vi "EditorEinfachPC.vi"() -> ()   [LabVIEW 2010]
panel:
  in  "EinstellungenSpeichern":bool
  out "Spannung Mach":fxp<+/-,16,4> format="%.14g"
  in  "Temperatur Mach":dbl
  out "Spannung Trap":fxp<+/-,16,4> format="%.14g"
  in  "Temperatur Trap":dbl
  out "LangsameHeizungen":string[](array[string])
  in  "AllesSpeichern":bool
  in  "ModuleLH":i32[](array[numeric]) min=1 max=3 step=1
  in  "NamenLangsameHeizungen":string[](array[string])
  out "Schnelle Heizungen":string[](array[string])
  in  "Modul3/AIsNamen":string[](array[string])
  in  "Modul2/AIsNamen":string[](array[string])
  in  "Modul1/AIsNamen":string[](array[string])
  out "Methoden":T1(array[cluster]) {"FPGAPID"."proportional gain (Kc)" format="%.11g"; "FPGAPID"."integral gain (Kc*Ts/Ti)" format="%.11g"; "FPGAPID"."derivative gain (Kc*Td/Ts)" format="%.11g"; "FPGAFixp" format="%.14g"}
  in  "Methodenname":string
  in  "Int.Stop2":dbl
  in  "Int.Start2":dbl
  in  "Int.Stop1":dbl
  in  "Int.Start1":dbl
  in  "ZeitpktMS-2":dbl
  in  "ZeitpktMS-1":dbl
  in  "SPMPV":i32[](array[numeric])
  in  "ZeitpunkteMPV":dbl[](array[numeric])
  in  "Regler für den Probenfluß":i32
  in  "DateinameECD2":string
  in  "DateiordnerECD2":path
  in  "DateinameECD1":string
  in  "DateiordnerECD1":path
  in  "Wert2":dbl
  in  "Vergleichsoperator2":dbl(ring) items=["<", "<=", "=", ">=", ">", "=/="]
  in  "AbfragbareVariablen2":dbl(ring) items=["T-Trap1", "T-Trap2", "T-Stirling", "T-PreCol1", "T-PreCol2", "T-MainCol1", "T-MainCol2", "T-MainCol3", "T-MainCol4", "T-Bronkh1", "T-Bronkh2", "T-Bronkh3", "T-Bronkh4", "T-Valve2", "T-Oven", "T-Valve1", "T-TransfLine", "T-TurboPump", "T-StirlingPlatine", "T-Spare3", "T-Spare4", "T-Spare5", "T-Spare6", "MFM1-1", "MFM1-2", "P-HighPress", "P-LowPress", "P-Vac", "TurboSpeed", "I-AC", "I-Trap1", "I-Trap2", "Mod2/AI0", "Mod2/AI1", "Mod2/AI2", "Mod2/AI3", "Mod2/AI4", "Mod2/AI5", "Mod2/AI6", "Mod2/AI7", "Mod2/AI8", "Mod2/AI9", "Mod2/AI10", "Mod2/AI11", "Mod2/AI12", "Mod2/AI13", "Mod2/AI14", "Mod2/AI15", "Mod2/AI16", "Mod2/AI17", "Mod2/AI18", "Mod2/AI19", "Mod2/AI20", "Mod2/AI21", "Mod2/AI22", "Mod2/AI23", "Mod2/AI24", "Mod2/AI25", "Mod2/AI26", "Mod2/AI27", "Mod2/AI28", "Mod2/AI29", "Mod2/AI30", "Mod2/AI31", "Mod3/AI0", "Mod3/AI1", "Mod3/AI2", "Mod3/AI3", "Mod3/AI4", "Mod3/AI5", "Mod3/AI6", "Mod3/AI7", "Mod3/AI8", "Mod3/AI9", "Mod3/AI10", "Mod3/AI11", "Mod3/AI12", "Mod3/AI13", "Mod3/AI14", "Mod3/AI15", "Mod3/AI16", "Mod3/AI17", "Mod3/AI18", "Mod3/AI19", "Mod3/AI20", "Mod3/AI21", "Mod3/AI22", "Mod3/AI23", "Mod3/AI24", "Mod3/AI25", "Mod3/AI26", "Mod3/AI27", "Mod3/AI28", "Mod3/AI29", "Mod3/AI30", "Mod3/AI31", "WiderstTrap1", "TempTrap1", "WiderstTrap2", "TempTrap2", "TempMach1", "TempMach2", "Regler18"]
  in  "Dateiname Housekeeping":string
  in  "Dateiordner Housekeeping":path=path "C:/Users/Atmos/Desktop/Johnny"
  in  "Startmethode":i32=1
  in  "Dateien fürs MS schicken?":bool
  in  "Zwangsbedingungen":dbl[][](array[numeric])
  out "ZwangsBedingungen":string[][](array[string])
  in  "löschen":bool
  in  "Bedingung Nr. X":i32
  in  "Bedingung übernehmen":bool
  in  "Ausgangswert":dbl
  in  "BedienbareVariablen":dbl(ring) items=["Mod5/DIO5", "Mod5/DIO6", "Mod5/DIO7", "Mod5/DIO10", "Mod5/DIO11", "Mod5/DIO14", "Mod5/DIO15", "Mod5/DIO16", "Mod5/DIO17", "Mod5/DIO18", "Mod5/DIO20", "Mod5/DIO23", "Mod5/DIO25", "Mod5/DIO26", "Mod5/DIO27", "Mod5/DIO28", "Mod5/DIO29", "Mod5/DIO30", "Mod6/DIO0", "Mod6/DIO1", "Mod6/DIO2", "Mod6/DIO3", "Mod6/DIO4", "Mod6/DIO5", "Mod6/DIO6", "Mod6/DIO7", "Mod6/DIO8", "Mod6/DIO9", "Mod6/DIO10", "Mod6/DIO11", "Mod6/DIO12", "Mod6/DIO13", "Mod6/DIO14", "Mod6/DIO15", "Mod6/DIO16", "Mod6/DIO17", "Mod6/DIO18", "Mod6/DIO19", "Mod6/DIO20", "Mod6/DIO21", "Mod6/DIO22", "Mod6/DIO23", "Mod6/DIO24", "Mod6/DIO25", "Mod6/DIO26", "Mod6/DIO27", "Mod6/DIO28", "Mod6/DIO29", "Mod6/DIO30", "Mod6/DIO31", "ServoTrap1kalt", "ServoTrap2kalt", "Heizen?Trap1", "Heizen?Trap2", "Heizen?Mach1", "Heizen?Mach2", "Methodennummer", "STOPP!!!", "LHHorst1Heizen?", "LHMainCol1Heizen?", "LHMainCol2Heizen?", "LHHorst2Heizen?", "LHOvenHeizen?", "LHT-LineHeizen?", "Regler18"]
  in  "Wert1":dbl
  in  "Vergleichsoperator1":dbl(ring) items=["<", "<=", "=", ">=", ">", "=/="]
  in  "AbfragbareVariablen1":dbl(ring) items=["T-Trap1", "T-Trap2", "T-Stirling", "T-PreCol1", "T-PreCol2", "T-MainCol1", "T-MainCol2", "T-MainCol3", "T-MainCol4", "T-Bronkh1", "T-Bronkh2", "T-Bronkh3", "T-Bronkh4", "T-Valve2", "T-Oven", "T-Valve1", "T-TransfLine", "T-TurboPump", "T-StirlingPlatine", "T-Spare3", "T-Spare4", "T-Spare5", "T-Spare6", "MFM1-1", "MFM1-2", "P-HighPress", "P-LowPress", "P-Vac", "TurboSpeed", "I-AC", "I-Trap1", "I-Trap2", "Mod2/AI0", "Mod2/AI1", "Mod2/AI2", "Mod2/AI3", "Mod2/AI4", "Mod2/AI5", "Mod2/AI6", "Mod2/AI7", "Mod2/AI8", "Mod2/AI9", "Mod2/AI10", "Mod2/AI11", "Mod2/AI12", "Mod2/AI13", "Mod2/AI14", "Mod2/AI15", "Mod2/AI16", "Mod2/AI17", "Mod2/AI18", "Mod2/AI19", "Mod2/AI20", "Mod2/AI21", "Mod2/AI22", "Mod2/AI23", "Mod2/AI24", "Mod2/AI25", "Mod2/AI26", "Mod2/AI27", "Mod2/AI28", "Mod2/AI29", "Mod2/AI30", "Mod2/AI31", "Mod3/AI0", "Mod3/AI1", "Mod3/AI2", "Mod3/AI3", "Mod3/AI4", "Mod3/AI5", "Mod3/AI6", "Mod3/AI7", "Mod3/AI8", "Mod3/AI9", "Mod3/AI10", "Mod3/AI11", "Mod3/AI12", "Mod3/AI13", "Mod3/AI14", "Mod3/AI15", "Mod3/AI16", "Mod3/AI17", "Mod3/AI18", "Mod3/AI19", "Mod3/AI20", "Mod3/AI21", "Mod3/AI22", "Mod3/AI23", "Mod3/AI24", "Mod3/AI25", "Mod3/AI26", "Mod3/AI27", "Mod3/AI28", "Mod3/AI29", "Mod3/AI30", "Mod3/AI31", "WiderstTrap1", "TempTrap1", "WiderstTrap2", "TempTrap2", "TempMach1", "TempMach2", "Regler18"]
  in  "AIsNamenZurücksetzen":bool
  in  "Methode Nummer":i32
  in  "MethodeLaden":bool
  in  "EditorBeenden":bool
  out "AnzahlRegler/Modul":i32[](array[numeric])
  in  "PIDs für \"träge\" Heizungen":T2(array[cluster])
  in  "AIsLH":i32[](array[numeric]) min=0 max=31 step=1
  in  "Traps/MachsKoeff":dbl[][](array[numeric])=[[0.0, 0.0, 0.0, 0.0, 0.0, 0.0, 0.0, 0.0, 0.0, 0.0, 0.0, 0.0, 0.0, 0.0, 0.0, 0.0, 0.0, 0.0, 0.0, 0.0, 0.0, 0.0, 0.0, 0.0, 0.0, 0.0, 0.0, 0.0, 0.0, 0.0, 0.0, 0.0]]
  in  "Modul3/AI koeff":dbl[][](array[numeric])=[[0.0, 0.0, 0.0, 0.0, 0.0, 0.0, 0.0, 0.0, 0.0, 0.0, 0.0, 0.0, 0.0, 0.0, 0.0, 0.0, 0.0, 0.0, 0.0, 0.0, 0.0, 0.0, 0.0, 0.0, 0.0, 0.0, 0.0, 0.0, 0.0, 0.0, 0.0, 0.0]]
  in  "Modul2/AI koeff":dbl[][](array[numeric])=[[0.0, 0.0, 0.0, 0.0, 0.0, 0.0, 0.0, 0.0, 0.0, 0.0, 0.0, 0.0, 0.0, 0.0, 0.0, 0.0, 0.0, 0.0, 0.0, 0.0, 0.0, 0.0, 0.0, 0.0, 0.0, 0.0, 0.0, 0.0, 0.0, 0.0, 0.0, 0.0]]
  in  "Modul1/AI koeff":dbl[][](array[numeric])=[[0.0, 0.0, 0.0, 0.0, 0.0, 0.0, 0.0, 0.0, 0.0, 0.0, 0.0, 0.0, 0.0, 0.0, 0.0, 0.0, 0.0, 0.0, 0.0, 0.0, 0.0, 0.0, 0.0, 0.0, 0.0, 0.0, 0.0, 0.0, 0.0, 0.0, 0.0, 0.0]]
  in  "TempMach2":dbl[](array[numeric])
  in  "ZeitpktMach2":dbl[](array[numeric])
  in  "TempMach1":dbl[](array[numeric])
  in  "ZeitpktMach1":dbl[](array[numeric])
  in  "FPGAFixp":fxp<+/-,16,4>[][](array[numeric]) format="%.14g"
  in  "ZeitpktFPGAFixp":dbl[](array[numeric])
  in  "FPGAPID":T3(array[cluster]) {"proportional gain (Kc)" format="%.11g"; "integral gain (Kc*Ts/Ti)" format="%.11g"; "derivative gain (Kc*Td/Ts)" format="%.11g"}
  in  "ZeitpktFPGAPID":dbl[](array[numeric])
  in  "FPGABoolesch":bool[][](array[boolean])
  in  "ZPktFPGABoolesch":dbl[](array[numeric])
  in  "LHHeizen?":bool[](array[boolean])
  in  "LHSetpoints":dbl[](array[numeric])
  out "HorstMod1Name":string[](array[string])
  out "HorstMod2AName":string[](array[string])
  out "HorstMod2BName":string[](array[string])
  in  "HorstSPMod1":dbl[][](array[numeric])
  in  "HorstSPMod2A":dbl[][](array[numeric])
  in  "HorstSPMod2B":dbl[][](array[numeric])
  in  "Mod1HorstZeitpkt":dbl[](array[numeric])
  in  "Mod2AHorstZeitpkt":dbl[](array[numeric])
  in  "Mod2BHorstZeitpkt":dbl[](array[numeric])
  in  "HorstSPMod0":dbl[][](array[numeric])
  out "HorstMod0Name":string[](array[string])
  in  "Mod0HorstZeitpkt":dbl[](array[numeric])
  in  "MWAntwortMod2B":string[](array[string])=[":060F020121", ":0610020121", ":0611020121"]
  in  "MWAntwortMod2A":string[](array[string])=[":060F020121", ":0610020121", ":0611020121"]
  in  "MWAntwortMod1":string[](array[string])=[":060F020121", ":0610020121", ":0611020121"]
  in  "MWAntwortMod0":string[](array[string])=[":060F020121", ":0610020121", ":0611020121"]
  in  "FaktorMod2B":dbl[](array[numeric])=[9.375e-05, 9.375e-05, 9.375e-05]
  in  "FaktorMod2A":dbl[](array[numeric])=[9.375e-05, 9.375e-05, 9.375e-05]
  in  "FaktorMod1":dbl[](array[numeric])=[9.375e-05, 9.375e-05, 9.375e-05]
  in  "FaktorMod0":dbl[](array[numeric])=[9.375e-05, 9.375e-05, 9.375e-05]
  in  "SPvorgebenMod2B":string[](array[string])=[":060F020121", ":0610020121", ":0611020121"]
  in  "SPvorgebenMod2A":string[](array[string])=[":060F020121", ":0610020121", ":0611020121"]
  in  "SPvorgebenMod1":string[](array[string])=[":060F020121", ":0610020121", ":0611020121"]
  in  "SPvorgebenMod0":string[](array[string])=[":060F020121", ":0610020121", ":0611020121"]
  in  "MWabfragenMod2B":string[](array[string])=[":060F0401210120", ":06100401210120", ":06110401210120"]
  in  "MWabfragenMod2A":string[](array[string])=[":060F0401210120", ":06100401210120", ":06110401210120"]
  in  "MWabfragenMod1":string[](array[string])=[":060F0401210120", ":06100401210120", ":06110401210120"]
  in  "MWabfragenMod0":string[](array[string])=[":060F0401210120", ":06100401210120", ":06110401210120"]
  in  "ReglerNameMod2B":string[](array[string])
  in  "ReglerNameMod2A":string[](array[string])
  in  "ReglerNameMod1":string[](array[string])
  in  "ReglerNameMod0":string[](array[string])
  in  "DIOsSPMod2B":bool[][](array[boolean])
  in  "DIOsSPMod2A":bool[][](array[boolean])
  in  "DIOsSPMod1":bool[][](array[boolean])
  in  "ZeitpktDIOsMod2B":dbl[](array[numeric])
  in  "ZeitpktDIOsMod2A":dbl[](array[numeric])
  in  "ZeitpktDIOsMod1":dbl[](array[numeric])
  out "DIOsMod2BName":string[](array[string])
  out "DIOsMod2AName":string[](array[string])
  out "DIOsMod1Name":string[](array[string])
  out "DIOsMod0Name":string[](array[string])
  in  "DIOsSPMod0":bool[][](array[boolean])
  in  "ZeitpktDIOsMod0":dbl[](array[numeric])
  in  "MethodeSpeichern":bool
  in  "EinstellungenFertig":bool
  in  "DIOsMod2BName":string[](array[string])
  in  "DIOsMod2AName":string[](array[string])
  in  "DIOsMod1Name":string[](array[string])
  in  "DIOsMod0Name":string[](array[string])
  in  "Zykluslängen [s]":dbl[](array[numeric])
  in  "DIOsMod2BNr":i32[](array[numeric]) min=0 max=63 step=1
  in  "DIOsMod2ANr":i32[](array[numeric]) min=0 max=63 step=1
  in  "DIOsMod1Nr":i32[](array[numeric]) min=0 max=63 step=1
  in  "DIOsMod0Nr":i32[](array[numeric]) min=0 max=63 step=1
  # "Hier gehts lang!"
  # "Hier gehts lang!"
  # "ServoTrap1 ServoTrap2  Heizen?      Heizen?      Heizen?      Heizen?\nkalt              kalt                Trap1          Trap2         Mach1        Mach2"
  # "Trap1"
  # "Trap2"
  # "Mach1"
  # "Mach2"
  # "Die Analogeingänge sind entsprechend der AI-Module des CRIO angeordnet (3x32); es wird eine quadratische Kennlinie angenommen, also: y=a0+a1*x+a2*x^2;\ndie drei Koeffizienten werden in dieser Reihenfolge eingegeben (v.l.n.r.): a0, a1, a2."
  # "Vorsicht!!! Wer hier nicht ganz genau weiß, was er tut, läßt bitte die Finger davon!\nDie Heizungen werden über den FPGA gesteuert, d.h. wenn man die Anzahl oder \ndie Anschlüsse der Heizungen ändert, muß das FPGA-Programm entsprechend\nangepaßt werden.\nModuleLH bezieht sich auf die drei AI-Module des CRIO (1,2,3) und AIsLH auf den\nAnschluß im jeweiligen Modul."
  # "Die digitalen Ein-/Ausgänge werden modulweise aufgelistet (0, 1, 2A, 2B) und benannt; die zugehörigen Anschlüsse\nwerden folgendermaßen durchgezählt: DIO 0...31 von Modul5 entspricht hier 0...31; DIO 0...31 von Modul6 entspricht hier 32+(0...31)=32...63."
  # "Im weiteren können beliebig viele Methoden definiert werden; mit welcher davon soll das Programm starten? Die erste Methode trägt die Nummer 0."
  # "Sososo... alle Einstellungen vorgenommen? Wirklich alle? Sicher? Bereit, mit den Methoden fortzufahren? Na super, dann trau Dich und drück den Knopf!"
  # "Es können beliebig viele Methoden definiert werden; die gewünschte Nummer auswählen und die entsprechende Methode laden, dann nach Belieben dran rumfummeln und anschließend, wenns beliebt, die vorgenommenen Änderungen an der Methode übernehmen (das bedeutet NICHT, daß die Änderungen in einer Datei abgelegt werden, dafür gibts nen extra Knopp);\n\"Editor beenden\" dürfte klar sein. Und Tschüß!"
  # ":::Tom \"Awesome\"  Burner Jr.:::"
  # "Sollen die Daten vom MS abgefragt werden? Wenn ja, zu welchen Zeitpunkten (im Zyklus1)?"
  # "Zur Erinnerung: die schnellen Heizungen regeln die Temperatur nur indirekt, die eigentliche Regelgröße ist die Spannung."
  # "Hier können direkt die Temperaturen vorgegeben werden, ohne den Umweg über die Spannung; die eingegebenen Punkte im (t-T)-Raum werden durch lineare Funktionen verbunden, jeweils definiert von Punkt zu Punkt."
  # "Stellung des Multipositionsventils; die Zeitpunkte beziehen sich auf den Zyklus von Modul0.\nDie Stellungen bezeichnen: \n1. Standard3 - 2. Luftprobe - 3. Blank - 4. Standard1 - 5. Standard2 - 6. nicht belegt"
  # "Innerhalb welcher Zeitfenster (Modul1) soll der Probenfluß integriert werden?"
  # "Der Gipfel der Flexibilität: die Zwangsbedingungen!\nBitte boolesche Werte als 0/1 eingeben"
  # "Dran denken: die Daten werden auf dem CRIO\nabgelegt, nicht auf dem Notebook;\nDateinamen bitte ohne Pfad und .tdms eingeben"
  # "Die Bronkhorst-Regler werden modulweise zusammengefasst an den CRIO \nangeschlossen, Mod0 an Port0, Mod1 an Port1, Mod2A&2B an Port2;\ndie Strings für die Steuerung und Abfrage der Regler ergeben sich aus dem bronkhorstschen Handbuch; der Faktor berechnet sich durch \"Vollausschlag des Reglers (in der gewünschten Einheit, z.B. Bar)\"/32000;\n'Regler für den Probenfluß' meint die Nummer des entsprechenden Reglers in der Liste aller Regler, wobei der erste die Nummer 0 trägt."
  # "Mod0\n\nMod1\n\nMod2A\n\nMod2B"
  # "UND"
  # "UTempSetpTrap1     UTempMaxTrap1     UWidrMaxTrap1      UTempSetpTrap2    UTempMaxTrap2    UWidrMaxTrap2      UMaxMach1             UMaxMach2"
types:
  T1 = cluster{"Zykluslängen [s]":dbl[], "ZeitpktDIOsMod0":dbl[], "ZeitpktDIOsMod1":dbl[], "ZeitpktDIOsMod2A":dbl[], "ZeitpktDIOsMod2B":dbl[], "DIOsSPMod0":bool[][], "DIOsSPMod1":bool[][], "DIOsSPMod2A":bool[][], "DIOsSPMod2B":bool[][], "Mod0HorstZeitpkt":dbl[], "Mod1HorstZeitpkt":dbl[], "Mod2AHorstZeitpkt":dbl[], "Mod2BHorstZeitpkt":dbl[], "HorstSPMod0":dbl[][], "HorstSPMod1":dbl[][], "HorstSPMod2A":dbl[][], "HorstSPMod2B":dbl[][], "LangsameHeizungenSP":dbl[], "LHHeizen?":bool[], "ZPktFPGABoolesch":dbl[], "FPGABoolesch":bool[][], "ZeitpktFPGAPID":dbl[], "FPGAPID":cluster{"proportional gain (Kc)":fxp<+/-,16,8>, "integral gain (Kc*Ts/Ti)":fxp<+/-,16,8>, "derivative gain (Kc*Td/Ts)":fxp<+/-,16,8>}[][], "ZeitpktFPGAFixp":dbl[], "FPGAFixp":fxp<+/-,16,4>[][], "ZeitpktMach1":dbl[], "TempMach1":dbl[], "ZeitpktMach2":dbl[], "TempMach2":dbl[], "PIDs für \"träge\" Heizungen":cluster{"proportional gain (Kc)":dbl, "integral time (Ti, min)":dbl, "derivative time (Td, min)":dbl}[], "Zwangsbedingungen":dbl[][], "Dateien fürs MS schicken?":bool, "ZeitpunkteMPV":dbl[], "SPMPV":i32[], "ZeitpktMSa":dbl, "ZeitpktMSb":dbl, "Int.Start1":dbl, "Int.Stop1":dbl, "Int.Start2":dbl, "Int.Stop2":dbl, "Methodenname":string}[]
  T2 = cluster{"proportional gain (Kc)":dbl, "integral time (Ti, min)":dbl, "derivative time (Td, min)":dbl}[]
  T3 = cluster{"proportional gain (Kc)":fxp<+/-,16,8>, "integral gain (Kc*Ts/Ti)":fxp<+/-,16,8>, "derivative gain (Kc*Td/Ts)":fxp<+/-,16,8>}[][]
  T4 = cluster{"DIOsMod0Nr":i32[], "DIOsMod1Nr":i32[], "DIOsMod2ANr":i32[], "DIOsMod2BNr":i32[], "AIsLH":i32[], "Anzahl Horst/Modul":i32[], "Regler für den Probenfluß":i32, "StringSPvorgebenMod0":string[], "StringSPvorgebenMod1":string[], "StringSPvorgebenMod2A":string[], "StringSPvorgebenMod2B":string[], "StringMWAntwort0":string[], "StringMWAntwort1":string[], "StringMWAntwort2A":string[], "StringMWAntwort2B":string[], "UmrechnungHorst0":dbl[], "UmrechnungHorst1":dbl[], "UmrechnungHorst2A":dbl[], "UmrechnungHorst2B":dbl[], "StringMWabfragenMod0":string[], "StringMWabfragenMod1":string[], "StringMWabfragenMod2A":string[], "StringMWabfragenMod2B":string[], "Modul1/AI koeff":dbl[][], "Modul2/AI koeff":dbl[][], "Modul3/AI koeff":dbl[][], "Traps/MachsKoeff":dbl[][], "Modul1/AIsNamen":string[], "Modul2/AIsNamen":string[], "Modul3/AIsNamen":string[], "DIOsMod0Name":string[], "DIOsMod1Name":string[], "DIOsMod2AName":string[], "DIOsMod2BName":string[], "HorstMod0Name":string[], "HorstMod1Name":string[], "HorstMod2AName":string[], "HorstMod2BName":string[], "Startmethode":i32, "Dateiordner Housekeeping":path, "Dateiname Housekeeping":string, "DateiordnerECD1":path, "DateinameECD1":string, "DateiordnerECD2":path, "DateinameECD2":string, "NamenLangsameHeizungen":string[], "ModuleLH":i32[]}
  T5 = cluster{"Zykluslängen [s]":dbl[], "ZeitpktDIOsMod0":dbl[], "ZeitpktDIOsMod1":dbl[], "ZeitpktDIOsMod2A":dbl[], "ZeitpktDIOsMod2B":dbl[], "DIOsSPMod0":bool[][], "DIOsSPMod1":bool[][], "DIOsSPMod2A":bool[][], "DIOsSPMod2B":bool[][], "Mod0HorstZeitpkt":dbl[], "Mod1HorstZeitpkt":dbl[], "Mod2AHorstZeitpkt":dbl[], "Mod2BHorstZeitpkt":dbl[], "HorstSPMod0":dbl[][], "HorstSPMod1":dbl[][], "HorstSPMod2A":dbl[][], "HorstSPMod2B":dbl[][], "LangsameHeizungenSP":dbl[], "LHHeizen?":bool[], "ZPktFPGABoolesch":dbl[], "FPGABoolesch":bool[][], "ZeitpktFPGAPID":dbl[], "FPGAPID":cluster{"proportional gain (Kc)":fxp<+/-,16,8>, "integral gain (Kc*Ts/Ti)":fxp<+/-,16,8>, "derivative gain (Kc*Td/Ts)":fxp<+/-,16,8>}[][], "ZeitpktFPGAFixp":dbl[], "FPGAFixp":fxp<+/-,16,4>[][], "ZeitpktMach1":dbl[], "TempMach1":dbl[], "ZeitpktMach2":dbl[], "TempMach2":dbl[], "PIDs für \"träge\" Heizungen":cluster{"proportional gain (Kc)":dbl, "integral time (Ti, min)":dbl, "derivative time (Td, min)":dbl}[], "Zwangsbedingungen":dbl[][], "Text0 MS-Datei":string, "Info":string, "wie wird gespeichert?":u16, "Speicherlänge":string, "Dateien fürs MS schicken?":bool, "Pfad MS-Datei CRIO":path}[]
  T6 = cluster{"DIOsMod0Nr":i32[], "DIOsMod1Nr":i32[], "DIOsMod2ANr":i32[], "DIOsMod2BNr":i32[], "AIs für \"träge\" Heizungen":i32[], i32[], "AnschlüsseHorstMod0":enum8{"0", "1", "2", "3", "4", "5", "6", "7", "8"}[], "AnschlüsseHorstMod1":enum8{"0", "1", "2", "3", "4", "5", "6", "7", "8"}[], "AnschlüsseHorstMod2A":enum8{"0", "1", "2", "3", "4", "5", "6", "7", "8"}[], "AnschlüsseHorstMod2B":enum8{"0", "1", "2", "3", "4", "5", "6", "7", "8"}[], "StringSPvorgebenMod0":string[], "StringSPvorgebenMod1":string[], "StringSPvorgebenMod2A":string[], "StringSPvorgebenMod2B":string[], "StringMWAntwort0":string[], "StringMWAntwort1":string[], "StringMWAntwort2A":string[], "StringMWAntwort2B":string[], "UmrechnungHorst0":dbl[], "UmrechnungHorst1":dbl[], "UmrechnungHorst2A":dbl[], "UmrechnungHorst2B":dbl[], "StringMWabfragenMod0":string[], "StringMWabfragenMod1":string[], "StringMWabfragenMod2A":string[], "StringMWabfragenMod2B":string[], "Modul1/AI koeff":dbl[][], "Modul2/AI koeff":dbl[][], "Modul3/AI koeff":dbl[][], "Traps/MachKoeff":dbl[][], "AIsNamen":string[], "DIOsMod0Name":string[], "DIOsMod1Name":string[], "DIOsMod2AName":string[], "DIOsMod2BName":string[], "HorstMod0Name":string[], "HorstMod1Name":string[], "HorstMod2AName":string[], "HorstMod2BName":string[], "Startmethode":i32, "Dateiordner Housekeeping":path, "Dateiname Housekeeping":string}
  T7 = enum16{"open", "replace", "create", "open or create", "replace or create", "replace or create with confirmation"}
  T8 = cluster{"DIOsMod0Nr":i32[], "DIOsMod1Nr":i32[], "DIOsMod2ANr":i32[], "DIOsMod2BNr":i32[], "AIsLH":i32[], "AnzahlRegler/Modul":i32[], "Regler für den Probenfluß":i32, "SPvorgebenMod0":string[], "SPvorgebenMod1":string[], "SPvorgebenMod2A":string[], "SPvorgebenMod2B":string[], "MWAntwortMod0":string[], "MWAntwortMod1":string[], "MWAntwortMod2A":string[], "MWAntwortMod2B":string[], "FaktorMod0":dbl[], "FaktorMod1":dbl[], "FaktorMod2A":dbl[], "FaktorMod2B":dbl[], "MWabfragenMod0":string[], "MWabfragenMod1":string[], "MWabfragenMod2A":string[], "MWabfragenMod2B":string[], "Modul1/AI koeff":dbl[][], "Modul2/AI koeff":dbl[][], "Modul3/AI koeff":dbl[][], "Traps/MachsKoeff":dbl[][], "Modul1/AIsNamen":string[], "Modul2/AIsNamen":string[], "Modul3/AIsNamen":string[], "DIOsMod0Name":string[], "DIOsMod1Name":string[], "DIOsMod2AName":string[], "DIOsMod2BName":string[], "ReglerNameMod0":string[], "ReglerNameMod1":string[], "ReglerNameMod2A":string[], "ReglerNameMod2B":string[], "Startmethode":i32, "Dateiordner Housekeeping":path, "Dateiname Housekeeping":string, "DateiordnerECD1":path, "DateinameECD1":string, "DateiordnerECD2":path, "DateinameECD2":string, "NamenLangsameHeizungen":string[], "ModuleLH":i32[]}
  T9 = cluster{"Zykluslängen [s]":dbl[], "ZeitpktDIOsMod0":dbl[], "ZeitpktDIOsMod1":dbl[], "ZeitpktDIOsMod2A":dbl[], "ZeitpktDIOsMod2B":dbl[], "DIOsSPMod0":bool[][], "DIOsSPMod1":bool[][], "DIOsSPMod2A":bool[][], "DIOsSPMod2B":bool[][], "Mod0HorstZeitpkt":dbl[], "Mod1HorstZeitpkt":dbl[], "Mod2AHorstZeitpkt":dbl[], "Mod2BHorstZeitpkt":dbl[], "HorstSPMod0":dbl[][], "HorstSPMod1":dbl[][], "HorstSPMod2A":dbl[][], "HorstSPMod2B":dbl[][], "LangsameHeizungenSP":dbl[], "LHHeizen?":bool[], "ZPktFPGABoolesch":dbl[], "FPGABoolesch":bool[][], "ZeitpktFPGAPID":dbl[], "FPGAPID":cluster{"proportional gain (Kc)":fxp<+/-,16,8>, "integral gain (Kc*Ts/Ti)":fxp<+/-,16,8>, "derivative gain (Kc*Td/Ts)":fxp<+/-,16,8>}[][], "ZeitpktFPGAFixp":dbl[], "FPGAFixp":fxp<+/-,16,4>[][], "ZeitpktMach1":dbl[], "TempMach1":dbl[], "ZeitpktMach2":dbl[], "TempMach2":dbl[], "PIDs für \"träge\" Heizungen":cluster{"proportional gain (Kc)":dbl, "integral time (Ti, min)":dbl, "derivative time (Td, min)":dbl}[], "Zwangsbedingungen":dbl[][], "Dateien fürs MS schicken?":bool, "ZeitpunkteMPV":dbl[], "SPMPV":i32[], "ZeitpktMSa":dbl, "ZeitpktMSb":dbl, "Int.Start1":dbl, "Int.Stop1":dbl, "Int.Start2":dbl, "Int.Stop2":dbl, "Methodenname":string}
  T10 = cluster{"Zykluslängen [s]":dbl[], "ZeitpktDIOsMod0":dbl[], "ZeitpktDIOsMod1":dbl[], "ZeitpktDIOsMod2A":dbl[], "ZeitpktDIOsMod2B":dbl[], "DIOsSPMod0":bool[][], "DIOsSPMod1":bool[][], "DIOsSPMod2A":bool[][], "DIOsSPMod2B":bool[][], "Mod0HorstZeitpkt":dbl[], "Mod1HorstZeitpkt":dbl[], "Mod2AHorstZeitpkt":dbl[], "Mod2BHorstZeitpkt":dbl[], "HorstSPMod0":dbl[][], "HorstSPMod1":dbl[][], "HorstSPMod2A":dbl[][], "HorstSPMod2B":dbl[][], "LHSetpoints":dbl[], "LHHeizen?":bool[], "ZPktFPGABoolesch":dbl[], "FPGABoolesch":bool[][], "ZeitpktFPGAPID":dbl[], "FPGAPID":cluster{"proportional gain (Kc)":fxp<+/-,16,8>, "integral gain (Kc*Ts/Ti)":fxp<+/-,16,8>, "derivative gain (Kc*Td/Ts)":fxp<+/-,16,8>}[][], "ZeitpktFPGAFixp":dbl[], "FPGAFixp":fxp<+/-,16,4>[][], "ZeitpktMach1":dbl[], "TempMach1":dbl[], "ZeitpktMach2":dbl[], "TempMach2":dbl[], "PIDs für \"träge\" Heizungen":cluster{"proportional gain (Kc)":dbl, "integral time (Ti, min)":dbl, "derivative time (Td, min)":dbl}[], "Zwangsbedingungen":dbl[][], "Dateien fürs MS schicken?":bool, "ZeitpunkteMPV":dbl[], "SPMPV":i32[], "ZeitpktMS-1":dbl, "ZeitpktMS-2":dbl, "Int.Start1":dbl, "Int.Stop1":dbl, "Int.Start2":dbl, "Int.Stop2":dbl, "Methodenname":string}
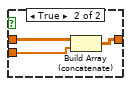
[diagram p7: hidden frame]
diagram:
  (unwired) T5 [{"Zykluslängen [s]"=[200.0, 200.0, 200.0, 200.0], "ZeitpktDIOsMod0"=[0.0, 200.0], "ZeitpktDIOsMod1"=[0.0, 1.0, 50.0, 60.0, 60.1, 70.0, 110.0, 200.0], "ZeitpktDIOsMod2A"=[0.0, 200.0], "ZeitpktDIOsMod2B"=[0.0, 60.0, 200.0], "DIOsSPMod0"=[[FALSE], [FALSE]], "DIOsSPMod1"=[[FALSE, TRUE, FALSE, TRUE, FALSE, TRUE, TRUE, FALSE, FALSE, FALSE, TRUE, TRUE, FALSE, FALSE, FALSE, FALSE, FALSE, TRUE], [FALSE, FALSE, FALSE, TRUE, FALSE, TRUE, TRUE, FALSE, FALSE, FALSE, TRUE, TRUE, FALSE, FALSE, FALSE, FALSE, FALSE, TRUE], [FALSE, FALSE, FALSE, FALSE, FALSE, TRUE, TRUE, FALSE, FALSE, FALSE, TRUE, FALSE, FALSE, FALSE, FALSE, FALSE, FALSE, TRUE], [FALSE, FALSE, FALSE, FALSE, FALSE, FALSE, TRUE, FALSE, FALSE, FALSE, TRUE, FALSE, FALSE, FALSE, FALSE, FALSE, FALSE, TRUE], [FALSE, FALSE, FALSE, FALSE, FALSE, FALSE, TRUE, FALSE, FALSE, FALSE, TRUE, FALSE, FALSE, FALSE, FALSE, FALSE, FALSE, TRUE], [FALSE, FALSE, FALSE, FALSE, FALSE, FALSE, TRUE, FALSE, FALSE, FALSE, TRUE, FALSE, FALSE, FALSE, FALSE, FALSE, FALSE, TRUE], [FALSE, FALSE, FALSE, FALSE, FALSE, FALSE, TRUE, FALSE, FALSE, FALSE, TRUE, FALSE, FALSE, FALSE, FALSE, FALSE, FALSE, TRUE], [FALSE, FALSE, FALSE, FALSE, FALSE, FALSE, TRUE, FALSE, FALSE, FALSE, TRUE, FALSE, FALSE, FALSE, FALSE, FALSE, FALSE, TRUE]], "DIOsSPMod2A"=[[FALSE], [FALSE]], "DIOsSPMod2B"=[[FALSE], [FALSE]], "Mod0HorstZeitpkt"=[0.0, 200.0], "Mod1HorstZeitpkt"=[0.0, 57.0, 72.0, 200.0], "Mod2AHorstZeitpkt"=[0.0, 60.0, 200.0], "Mod2BHorstZeitpkt"=[0.0, 200.0], "HorstSPMod0"=[[2.6], [2.6]], "HorstSPMod1"=[[1.6, 0.0, 1.3], [0.0, 0.0, 1.3], [1.6, 0.0, 1.3], [1.6, 0.0, 1.3]], "HorstSPMod2A"=[[500.0], [0.0], [0.0]], "HorstSPMod2B"=[[0.0], [0.0]], "LangsameHeizungenSP"=[60.0, 200.0, 220.0, 60.0, 90.0, 0.0], "LHHeizen?"=[FALSE, FALSE, FALSE, FALSE, FALSE, FALSE], "ZPktFPGABoolesch"=[0.0, 60.0, 80.0, 200.0], "FPGABoolesch"=[[FALSE, FALSE, FALSE, FALSE, TRUE, FALSE], [FALSE, FALSE, TRUE, FALSE, TRUE, FALSE], [FALSE, FALSE, FALSE, FALSE, TRUE, FALSE], [FALSE, FALSE, FALSE, FALSE, TRUE, FALSE]], "ZeitpktFPGAPID"=[0.0, 60.0, 200.0], "FPGAPID"=[[{"proportional gain (Kc)"=2.0, "integral gain (Kc*Ts/Ti)"=1.66796875, "derivative gain (Kc*Td/Ts)"=0.0}, {"proportional gain (Kc)"=1.0, "integral gain (Kc*Ts/Ti)"=1.66796875, "derivative gain (Kc*Td/Ts)"=0.0}, {"proportional gain (Kc)"=5.0, "integral gain (Kc*Ts/Ti)"=0.03515625, "derivative gain (Kc*Td/Ts)"=0.0234375}, {"proportional gain (Kc)"=1.0, "integral gain (Kc*Ts/Ti)"=1.66796875, "derivative gain (Kc*Td/Ts)"=0.0}], [{"proportional gain (Kc)"=2.0, "integral gain (Kc*Ts/Ti)"=1.66796875, "derivative gain (Kc*Td/Ts)"=0.0}, {"proportional gain (Kc)"=1.0, "integral gain (Kc*Ts/Ti)"=1.66796875, "derivative gain (Kc*Td/Ts)"=0.0}, {"proportional gain (Kc)"=5.0, "integral gain (Kc*Ts/Ti)"=0.03515625, "derivative gain (Kc*Td/Ts)"=0.0234375}, {"proportional gain (Kc)"=1.0, "integral gain (Kc*Ts/Ti)"=1.66796875, "derivative gain (Kc*Td/Ts)"=0.0}], [{"proportional gain (Kc)"=0.0, "integral gain (Kc*Ts/Ti)"=0.0, "derivative gain (Kc*Td/Ts)"=0.0}, {"proportional gain (Kc)"=0.0, "integral gain (Kc*Ts/Ti)"=0.0, "derivative gain (Kc*Td/Ts)"=0.0}, {"proportional gain (Kc)"=5.0, "integral gain (Kc*Ts/Ti)"=0.03125, "derivative gain (Kc*Td/Ts)"=0.01953125}, {"proportional gain (Kc)"=0.0, "integral gain (Kc*Ts/Ti)"=0.0, "derivative gain (Kc*Td/Ts)"=0.0}], [{"proportional gain (Kc)"=0.0, "integral gain (Kc*Ts/Ti)"=0.0, "derivative gain (Kc*Td/Ts)"=0.0}, {"proportional gain (Kc)"=0.0, "integral gain (Kc*Ts/Ti)"=0.0, "derivative gain (Kc*Td/Ts)"=0.0}, {"proportional gain (Kc)"=5.0, "integral gain (Kc*Ts/Ti)"=0.03125, "derivative gain (Kc*Td/Ts)"=0.01953125}, {"proportional gain (Kc)"=0.0, "integral gain (Kc*Ts/Ti)"=0.0, "derivative gain (Kc*Td/Ts)"=0.0}], [{"proportional gain (Kc)"=0.0, "integral gain (Kc*Ts/Ti)"=0.0, "derivative gain (Kc*Td/Ts)"=0.0}, {"proportional gain (Kc)"=0.0, "integral gain (Kc*Ts/Ti)"=0.0, "derivative gain (Kc*Td/Ts)"=0.0}, {"proportional gain (Kc)"=5.0, "integral gain (Kc*Ts/Ti)"=0.03125, "derivative gain (Kc*Td/Ts)"=0.01953125}, {"proportional gain (Kc)"=0.0, "integral gain (Kc*Ts/Ti)"=0.0, "derivative gain (Kc*Td/Ts)"=0.0}]], "ZeitpktFPGAFixp"=[0.0, 61.0, 70.0, 200.0], "FPGAFixp"=[[0.0, 0.0, 0.0, 0.0, 0.0, 0.0, 2.60009765625, 0.0], [4.199951171875, 4.199951171875, 1.75, 0.0, 0.0, 0.0, 2.60009765625, 0.0], [0.0, 0.0, 0.0, 0.0, 0.0, 0.0, 2.60009765625, 0.0], [0.0, 0.0, 0.0, 0.0, 0.0, 0.0, 2.60009765625, 0.0]], "ZeitpktMach1"=[0.0, 80.0, 85.0, 119.0, 200.0], "TempMach1"=[30.0, 30.0, 220.0, 220.0, 30.0], "ZeitpktMach2"=[0.0, 0.0, 120.0], "TempMach2"=[0.0, 0.0, 0.0], "PIDs für \"träge\" Heizungen"=[{"proportional gain (Kc)"=1.0, "integral time (Ti, min)"=0.01, "derivative time (Td, min)"=0.0}, {"proportional gain (Kc)"=4.0, "integral time (Ti, min)"=1.0, "derivative time (Td, min)"=0.0}, {"proportional gain (Kc)"=4.0, "integral time (Ti, min)"=1.0, "derivative time (Td, min)"=0.0}, {"proportional gain (Kc)"=1.0, "integral time (Ti, min)"=0.01, "derivative time (Td, min)"=0.0}, {"proportional gain (Kc)"=2.0, "integral time (Ti, min)"=0.0, "derivative time (Td, min)"=0.0}, {"proportional gain (Kc)"=1.0, "integral time (Ti, min)"=0.01, "derivative time (Td, min)"=0.0}], "Zwangsbedingungen"=[[3.0, 4.0, 100.0, 23.0, 4.0, 200.0, 0.0, 0.0]], "Text0 MS-Datei"="text0", "Info"="info", "wie wird gespeichert?"=0, "Speicherlänge"="100", "Dateien fürs MS schicken?"=FALSE, "Pfad MS-Datei CRIO"=path "c:/"}] ("Zykluszeug 2")
  (unwired) T5 [{"Zykluslängen [s]"=[180.0, 180.0, 180.0, 180.0], "ZeitpktDIOsMod0"=[0.0, 180.0], "ZeitpktDIOsMod1"=[0.0, 1.0, 56.0, 60.0, 60.1, 70.0, 110.0, 180.0], "ZeitpktDIOsMod2A"=[0.0, 180.0], "ZeitpktDIOsMod2B"=[0.0, 60.0, 180.0], "DIOsSPMod0"=[[FALSE], [FALSE]], "DIOsSPMod1"=[[TRUE, TRUE, FALSE, TRUE, FALSE, TRUE, TRUE, FALSE, FALSE, FALSE, TRUE, TRUE, FALSE, TRUE, FALSE, FALSE, FALSE, TRUE], [TRUE, FALSE, FALSE, TRUE, FALSE, TRUE, TRUE, FALSE, FALSE, FALSE, TRUE, TRUE, FALSE, TRUE, FALSE, FALSE, FALSE, TRUE], [TRUE, FALSE, FALSE, FALSE, FALSE, TRUE, TRUE, FALSE, FALSE, FALSE, TRUE, FALSE, FALSE, TRUE, FALSE, FALSE, FALSE, TRUE], [TRUE, FALSE, FALSE, FALSE, FALSE, FALSE, TRUE, FALSE, FALSE, FALSE, TRUE, FALSE, FALSE, TRUE, FALSE, FALSE, FALSE, TRUE], [TRUE, FALSE, FALSE, FALSE, FALSE, FALSE, TRUE, FALSE, FALSE, FALSE, TRUE, FALSE, FALSE, TRUE, FALSE, FALSE, FALSE, TRUE], [TRUE, FALSE, FALSE, FALSE, FALSE, FALSE, TRUE, FALSE, FALSE, FALSE, TRUE, FALSE, FALSE, TRUE, FALSE, FALSE, FALSE, TRUE], [TRUE, FALSE, FALSE, TRUE, FALSE, FALSE, TRUE, FALSE, FALSE, FALSE, TRUE, FALSE, FALSE, TRUE, FALSE, FALSE, FALSE, TRUE], [TRUE, FALSE, FALSE, TRUE, FALSE, FALSE, TRUE, FALSE, FALSE, FALSE, TRUE, FALSE, FALSE, TRUE, FALSE, FALSE, FALSE, TRUE]], "DIOsSPMod2A"=[[FALSE], [FALSE]], "DIOsSPMod2B"=[[FALSE], [FALSE]], "Mod0HorstZeitpkt"=[0.0, 180.0], "Mod1HorstZeitpkt"=[0.0, 57.0, 72.0, 180.0], "Mod2AHorstZeitpkt"=[0.0, 60.0, 180.0], "Mod2BHorstZeitpkt"=[0.0, 120.0], "HorstSPMod0"=[[2.6], [2.6]], "HorstSPMod1"=[[1.6, 0.0, 1.3], [0.0, 0.0, 1.3], [1.6, 0.0, 1.3], [1.6, 0.0, 1.3]], "HorstSPMod2A"=[[500.0], [0.0], [0.0]], "HorstSPMod2B"=[[0.0], [0.0]], "LangsameHeizungenSP"=[60.0, 220.0, 220.0, 60.0, 70.0, 0.0], "LHHeizen?"=[TRUE, TRUE, TRUE, TRUE, TRUE, FALSE], "ZPktFPGABoolesch"=[0.0, 61.0, 80.0, 180.0], "FPGABoolesch"=[[FALSE, FALSE, FALSE, FALSE, TRUE, FALSE], [FALSE, FALSE, TRUE, FALSE, TRUE, FALSE], [FALSE, FALSE, FALSE, FALSE, TRUE, FALSE], [FALSE, FALSE, FALSE, FALSE, TRUE, FALSE]], "ZeitpktFPGAPID"=[0.0, 60.0, 180.0], "FPGAPID"=[[{"proportional gain (Kc)"=1.0, "integral gain (Kc*Ts/Ti)"=1.66796875, "derivative gain (Kc*Td/Ts)"=0.0}, {"proportional gain (Kc)"=1.0, "integral gain (Kc*Ts/Ti)"=1.66796875, "derivative gain (Kc*Td/Ts)"=0.0}, {"proportional gain (Kc)"=5.0, "integral gain (Kc*Ts/Ti)"=0.03515625, "derivative gain (Kc*Td/Ts)"=0.0234375}, {"proportional gain (Kc)"=1.0, "integral gain (Kc*Ts/Ti)"=1.66796875, "derivative gain (Kc*Td/Ts)"=0.0}], [{"proportional gain (Kc)"=1.0, "integral gain (Kc*Ts/Ti)"=1.66796875, "derivative gain (Kc*Td/Ts)"=0.0}, {"proportional gain (Kc)"=1.0, "integral gain (Kc*Ts/Ti)"=1.66796875, "derivative gain (Kc*Td/Ts)"=0.0}, {"proportional gain (Kc)"=5.0, "integral gain (Kc*Ts/Ti)"=0.03515625, "derivative gain (Kc*Td/Ts)"=0.0234375}, {"proportional gain (Kc)"=1.0, "integral gain (Kc*Ts/Ti)"=1.66796875, "derivative gain (Kc*Td/Ts)"=0.0}], [{"proportional gain (Kc)"=0.0, "integral gain (Kc*Ts/Ti)"=0.0, "derivative gain (Kc*Td/Ts)"=0.0}, {"proportional gain (Kc)"=0.0, "integral gain (Kc*Ts/Ti)"=0.0, "derivative gain (Kc*Td/Ts)"=0.0}, {"proportional gain (Kc)"=5.0, "integral gain (Kc*Ts/Ti)"=0.03125, "derivative gain (Kc*Td/Ts)"=0.01953125}, {"proportional gain (Kc)"=0.0, "integral gain (Kc*Ts/Ti)"=0.0, "derivative gain (Kc*Td/Ts)"=0.0}], [{"proportional gain (Kc)"=0.0, "integral gain (Kc*Ts/Ti)"=0.0, "derivative gain (Kc*Td/Ts)"=0.0}, {"proportional gain (Kc)"=0.0, "integral gain (Kc*Ts/Ti)"=0.0, "derivative gain (Kc*Td/Ts)"=0.0}, {"proportional gain (Kc)"=5.0, "integral gain (Kc*Ts/Ti)"=0.03125, "derivative gain (Kc*Td/Ts)"=0.01953125}, {"proportional gain (Kc)"=0.0, "integral gain (Kc*Ts/Ti)"=0.0, "derivative gain (Kc*Td/Ts)"=0.0}], [{"proportional gain (Kc)"=0.0, "integral gain (Kc*Ts/Ti)"=0.0, "derivative gain (Kc*Td/Ts)"=0.0}, {"proportional gain (Kc)"=0.0, "integral gain (Kc*Ts/Ti)"=0.0, "derivative gain (Kc*Td/Ts)"=0.0}, {"proportional gain (Kc)"=5.0, "integral gain (Kc*Ts/Ti)"=0.03125, "derivative gain (Kc*Td/Ts)"=0.01953125}, {"proportional gain (Kc)"=0.0, "integral gain (Kc*Ts/Ti)"=0.0, "derivative gain (Kc*Td/Ts)"=0.0}]], "ZeitpktFPGAFixp"=[0.0, 61.0, 70.0, 180.0], "FPGAFixp"=[[0.0, 0.0, 0.0, 0.0, 0.0, 0.0, 2.60009765625, 0.0], [4.199951171875, 4.199951171875, 1.800048828125, 0.0, 0.0, 0.0, 2.60009765625, 0.0], [0.0, 0.0, 0.0, 0.0, 0.0, 0.0, 2.60009765625, 0.0], [0.0, 0.0, 0.0, 0.0, 0.0, 0.0, 2.60009765625, 0.0]], "ZeitpktMach1"=[0.0, 75.0, 80.0, 150.0, 151.0, 180.0], "TempMach1"=[30.0, 30.0, 220.0, 220.0, 30.0, 30.0], "ZeitpktMach2"=[0.0, 0.0, 120.0], "TempMach2"=[0.0, 0.0, 0.0], "PIDs für \"träge\" Heizungen"=[{"proportional gain (Kc)"=1.0, "integral time (Ti, min)"=0.01, "derivative time (Td, min)"=0.0}, {"proportional gain (Kc)"=4.0, "integral time (Ti, min)"=1.0, "derivative time (Td, min)"=0.0}, {"proportional gain (Kc)"=4.0, "integral time (Ti, min)"=1.0, "derivative time (Td, min)"=0.0}, {"proportional gain (Kc)"=1.0, "integral time (Ti, min)"=0.01, "derivative time (Td, min)"=0.0}, {"proportional gain (Kc)"=2.0, "integral time (Ti, min)"=0.0, "derivative time (Td, min)"=0.0}, {"proportional gain (Kc)"=1.0, "integral time (Ti, min)"=0.01, "derivative time (Td, min)"=0.0}], "Zwangsbedingungen"=[[0.0, 0.0, 0.0, 0.0, 0.0]], "Text0 MS-Datei"="text0", "Info"="info", "wie wird gespeichert?"=0, "Speicherlänge"="100", "Dateien fürs MS schicken?"=FALSE, "Pfad MS-Datei CRIO"=path "c:/"}] ("Eingang")
  (unwired) T6 {"DIOsMod0Nr"=[32], "DIOsMod1Nr"=[5, 6, 7, 10, 11, 14, 15, 16, 17, 18, 20, 23, 25, 26, 27, 28, 29, 30], "DIOsMod2ANr"=[33], "DIOsMod2BNr"=[34], "AIs für \"träge\" Heizungen"=[17, 6, 0, 19, 21, 23], [1, 3, 1, 1], "AnschlüsseHorstMod0"=[enum."1"], "AnschlüsseHorstMod1"=[enum."1", enum."1", enum."1"], "AnschlüsseHorstMod2A"=[enum."1"], "AnschlüsseHorstMod2B"=[enum."1"], "StringSPvorgebenMod0"=[":060A020121"], "StringSPvorgebenMod1"=[":060B020121", ":0618020121", ":060D020121"], "StringSPvorgebenMod2A"=[":0619020121"], "StringSPvorgebenMod2B"=[":060C020121"], "StringMWAntwort0"=[":060A020121"], "StringMWAntwort1"=[":060B020121", ":0618020121", ":060D020121"], "StringMWAntwort2A"=[":0619020121"], "StringMWAntwort2B"=[":060C020121"], "UmrechnungHorst0"=[0.0003125], "UmrechnungHorst1"=[9.375e-05, 9.375e-05, 9.375e-05], "UmrechnungHorst2A"=[0.046875], "UmrechnungHorst2B"=[9.375e-05], "StringMWabfragenMod0"=[":060A0401210120"], "StringMWabfragenMod1"=[":060B0401210120", ":06180401210120", ":060D0401210120"], "StringMWabfragenMod2A"=[":06190401210120"], "StringMWabfragenMod2B"=[":060C0401210120"], "Modul1/AI koeff"=[[-249.333, 111.873, 2.1471], [-249.333, 111.873, 2.1471], [-249.333, 111.873, 2.1471], [-249.333, 111.873, 2.1471], [-237.2852, -153.162, 6.0782], [-237.2852, -153.162, 6.0782], [-249.333, 111.873, 2.1471], [-249.333, 111.873, 2.1471], [-249.333, 111.873, 2.1471], [-249.333, 111.873, 2.1471], [-249.333, 111.873, 2.1471], [-249.333, 111.873, 2.1471], [-249.333, 111.873, 2.1471], [-249.333, 111.873, 2.1471], [-249.333, 111.873, 2.1471], [0.0, 1.0, 0.0], [-249.333, 111.873, 2.1471], [-249.333, 111.873, 2.1471], [-249.333, 111.873, 2.1471], [-249.333, 111.873, 2.1471], [-249.333, 111.873, 2.1471], [-249.333, 111.873, 2.1471], [-249.333, 111.873, 2.1471], [-249.333, 111.873, 2.1471], [0.0, 1.0, 0.0], [0.0, 1.0, 0.0], [0.0, 1.0, 0.0], [0.0, 1.0, 0.0], [0.0, 1.0, 0.0], [0.0, 1.0, 0.0], [0.0, 1.0, 0.0], [0.0, 1.0, 0.0]], "Modul2/AI koeff"=[[0.0, 1.0, 0.0], [0.0, 1.0, 0.0], [0.0, 1.0, 0.0], [0.0, 1.0, 0.0], [0.0, 1.0, 0.0], [0.0, 1.0, 0.0], [0.0, 1.0, 0.0], [0.0, 1.0, 0.0], [0.0, 1.0, 0.0], [0.0, 1.0, 0.0], [0.0, 1.0, 0.0], [0.0, 1.0, 0.0], [0.0, 1.0, 0.0], [0.0, 1.0, 0.0], [0.0, 1.0, 0.0], [0.0, 1.0, 0.0], [0.0, 1.0, 0.0], [0.0, 1.0, 0.0], [0.0, 1.0, 0.0], [0.0, 1.0, 0.0], [0.0, 1.0, 0.0], [0.0, 1.0, 0.0], [0.0, 1.0, 0.0], [0.0, 1.0, 0.0], [0.0, 1.0, 0.0], [0.0, 1.0, 0.0], [0.0, 1.0, 0.0], [0.0, 1.0, 0.0], [0.0, 1.0, 0.0], [0.0, 1.0, 0.0], [0.0, 1.0, 0.0], [0.0, 1.0, 0.0]], "Modul3/AI koeff"=[[0.0, 1.0, 0.0], [0.0, 1.0, 0.0], [0.0, 1.0, 0.0], [0.0, 1.0, 0.0], [0.0, 1.0, 0.0], [0.0, 1.0, 0.0], [0.0, 1.0, 0.0], [0.0, 1.0, 0.0], [0.0, 1.0, 0.0], [0.0, 1.0, 0.0], [0.0, 1.0, 0.0], [0.0, 1.0, 0.0], [0.0, 1.0, 0.0], [0.0, 1.0, 0.0], [0.0, 1.0, 0.0], [0.0, 1.0, 0.0], [0.0, 1.0, 0.0], [0.0, 1.0, 0.0], [0.0, 1.0, 0.0], [0.0, 1.0, 0.0], [0.0, 1.0, 0.0], [0.0, 1.0, 0.0], [0.0, 1.0, 0.0], [0.0, 1.0, 0.0], [0.0, 1.0, 0.0], [0.0, 1.0, 0.0], [0.0, 1.0, 0.0], [0.0, 1.0, 0.0], [0.0, 1.0, 0.0], [0.0, 1.0, 0.0], [0.0, 1.0, 0.0], [0.0, 1.0, 0.0]], "Traps/MachKoeff"=[[0.0, 1.0, 0.0], [-249.333, 111.873, 2.1471], [0.0, 1.0, 0.0], [-249.333, 111.873, 2.1471], [-237.2852, 153.1621, 6.0782], [-237.2852, 153.1621, 6.0782]], "AIsNamen"=["T-MainCol3", "T-Trap1", "T-Trap2", "T-Stirling", "T-PreCol1", "T-PreCol2", "T-MainCol1", "T-MainCol2", "T-T-Line2", "T-MI1", "T-MI2", "T-MI3", "T-MI4", "T-MI5", "T-MI6", "F-MFM1", "T-MainCol4", "T-BHorst1", "T-BHorst2", "T-BHorst3", "T-BHorst4", "T-Oven1", "T-Oven2", "T-T-Line1", "F-MFM2", "P-Me-HP", "P-Me-LP", "P-Vac", "Ref-Turbo", "I-MS-AC", "I-Trap1", "I-Trap2", "Mod2/AI0", "Mod2/AI1", "Mod2/AI2", "Mod2/AI3", "Mod2/AI4", "Mod2/AI5", "Mod2/AI6", "Mod2/AI7", "Mod2/AI8", "Mod2/AI9", "Mod2/AI10", "Mod2/AI11", "Mod2/AI12", "Mod2/AI13", "Mod2/AI14", "Mod2/AI15", "Mod2/AI16", "Mod2/AI17", "Mod2/AI18", "Mod2/AI19", "Mod2/AI20", "Mod2/AI21", "Mod2/AI22", "Mod2/AI23", "Mod2/AI24", "Mod2/AI25", "Mod2/AI26", "Mod2/AI27", "Mod2/AI28", "Mod2/AI29", "Mod2/AI30", "Mod2/AI31", "Mod3/AI0", "Mod3/AI1", "Mod3/AI2", "Mod3/AI3", "Mod3/AI4", "Mod3/AI5", "Mod3/AI6", "Mod3/AI7", "Mod3/AI8", "Mod3/AI9", "Mod3/AI10", "Mod3/AI11", "Mod3/AI12", "Mod3/AI13", "Mod3/AI14", "Mod3/AI15", "Mod3/AI16", "Mod3/AI17", "Mod3/AI18", "Mod3/AI19", "Mod3/AI20", "Mod3/AI21", "Mod3/AI22", "Mod3/AI23", "Mod3/AI24", "Mod3/AI25", "Mod3/AI26", "Mod3/AI27", "Mod3/AI28", "Mod3/AI29", "Mod3/AI30", "Mod3/AI31"], "DIOsMod0Name"=["blindDIO0"], "DIOsMod1Name"=["on/off P-MS", "MS Start", "MS Stop", "FanMach1", "FanReserve", "Valve1A", "on/off PrePump", "S1Reserve", "on/off VacP2", "on/off VacP1", "S1D", "FanMach2", "S1C", "on/off Stirling", "S1B", "S1A", "Valve1B", "on/off Turbo"], "DIOsMod2AName"=["blindDIO2A"], "DIOsMod2BName"=["blindDIO2B"], "HorstMod0Name"=["MFC1B"], "HorstMod1Name"=["PressContr1A", "PressContr1B", "PressContr1C"], "HorstMod2AName"=["MFC1A"], "HorstMod2BName"=["PressContr1D"], "Startmethode"=0, "Dateiordner Housekeeping"=path "C:/", "Dateiname Housekeeping"="test"} ("Einstellungen 2")
  n1 = Open/Create/Replace File(file path (use dialog)=path "c:/einstellungen.per" ("Dateipfad Einstellungen")) -> (refnum out=w16:refnum<file>, error out=w17:errorcluster)  [unwired: 5 in, 1 out]
  n2 = Read from Binary File(5:T4 {"DIOsMod0Nr"=[], "DIOsMod1Nr"=[], "DIOsMod2ANr"=[], "DIOsMod2BNr"=[], "AIsLH"=[], "Anzahl Horst/Modul"=[], "Regler für den Probenfluß"=0, "StringSPvorgebenMod0"=[], "StringSPvorgebenMod1"=[], "StringSPvorgebenMod2A"=[], "StringSPvorgebenMod2B"=[], "StringMWAntwort0"=[], "StringMWAntwort1"=[], "StringMWAntwort2A"=[], "StringMWAntwort2B"=[], "UmrechnungHorst0"=[], "UmrechnungHorst1"=[], "UmrechnungHorst2A"=[], "UmrechnungHorst2B"=[], "StringMWabfragenMod0"=[], "StringMWabfragenMod1"=[], "StringMWabfragenMod2A"=[], "StringMWabfragenMod2B"=[], "Modul1/AI koeff"=[], "Modul2/AI koeff"=[], "Modul3/AI koeff"=[], "Traps/MachsKoeff"=[], "Modul1/AIsNamen"=[], "Modul2/AIsNamen"=[], "Modul3/AIsNamen"=[], "DIOsMod0Name"=[], "DIOsMod1Name"=[], "DIOsMod2AName"=[], "DIOsMod2BName"=[], "HorstMod0Name"=[], "HorstMod1Name"=[], "HorstMod2AName"=[], "HorstMod2BName"=[], "Startmethode"=0, "Dateiordner Housekeeping"=path "", "Dateiname Housekeeping"="", "DateiordnerECD1"=path "", "DateinameECD1"="", "DateiordnerECD2"=path "", "DateinameECD2"="", "NamenLangsameHeizungen"=[], "ModuleLH"=[]} ("Einstellungen"), 8:w17, 11:w16) -> (0:w12:errorcluster, 2:w14:T4, 3:w13:refnum<file>)  [unwired: 3 in, 1 out]
  n3 = Close File(refnum=w13, error in=w12) -> (path=w10:path, error out=w11:errorcluster)
  n4 = call <vilib>:"Simple Error Handler.vi"("error in (no error)"=w11) -> ()  [unwired: 4 in, 5 out]
  n5 = flat-sequence {
    tunnel: w14 -> [w82]
    tunnel: [w102] -> w33
    tunnel: [w101] -> w32
    tunnel: [w100] -> w31
    tunnel: [w99] -> w30
    tunnel: [w98] -> w29
    tunnel: [w97] -> w28
    tunnel: [w96] -> w27
    tunnel: [w95] -> w26
    tunnel: [w94] -> w25
    tunnel: [w89] -> w24
    tunnel: [w88] -> w23
    tunnel: [w87] -> w22
    tunnel: [w86] -> w21
    tunnel: [w85] -> w20
    tunnel: [w84] -> w19
    tunnel: w10 -> [w83]
    tunnel: w33 -> [w203]
    tunnel: w32 -> [w202]
    tunnel: w31 -> [w201]
    tunnel: w30 -> [w200]
    tunnel: w29 -> [w199]
    tunnel: w28 -> [w198]
    tunnel: w27 -> [w196]
    tunnel: w26 -> [w197]
    tunnel: w25 -> [w195]
    tunnel: w24 -> [w186]
    tunnel: w23 -> [w193]
    tunnel: w22 -> [w192]
    tunnel: w21 -> [w191]
    tunnel: w20 -> [w190]
    tunnel: w6 -> [w189]
    tunnel: w19 -> [w181]
    tunnel: w1 -> [w180]
    frame #0 {
      n6 = Unbundle(w82) -> ("DIOsMod0Nr"=w81:i32[], "DIOsMod1Nr"=w80:i32[], "DIOsMod2ANr"=w79:i32[], "DIOsMod2BNr"=w78:i32[], "AIsLH"=w77:i32[], "Anzahl Horst/Modul"=w76:i32[], "Regler für den Probenfluß"=w75:i32, "StringSPvorgebenMod0"=w74:string[], "StringSPvorgebenMod1"=w73:string[], "StringSPvorgebenMod2A"=w72:string[], "StringSPvorgebenMod2B"=w71:string[], "StringMWAntwort0"=w70:string[], "StringMWAntwort1"=w69:string[], "StringMWAntwort2A"=w68:string[], "StringMWAntwort2B"=w67:string[], "UmrechnungHorst0"=w66:dbl[], "UmrechnungHorst1"=w65:dbl[], "UmrechnungHorst2A"=w64:dbl[], "UmrechnungHorst2B"=w63:dbl[], "StringMWabfragenMod0"=w62:string[], "StringMWabfragenMod1"=w61:string[], "StringMWabfragenMod2A"=w60:string[], "StringMWabfragenMod2B"=w59:string[], "Modul1/AI koeff"=w58:dbl[][], "Modul2/AI koeff"=w57:dbl[][], "Modul3/AI koeff"=w56:dbl[][], "Traps/MachsKoeff"=w55:dbl[][], "Modul1/AIsNamen"=w54:string[], "Modul2/AIsNamen"=w53:string[], "Modul3/AIsNamen"=w52:string[], "DIOsMod0Name"=w51:string[], "DIOsMod1Name"=w50:string[], "DIOsMod2AName"=w49:string[], "DIOsMod2BName"=w48:string[], "HorstMod0Name"=w47:string[], "HorstMod1Name"=w46:string[], "HorstMod2AName"=w45:string[], "HorstMod2BName"=w44:string[], "Startmethode"=w43:i32, "Dateiordner Housekeeping"=w42:path, "Dateiname Housekeeping"=w41:string, "DateiordnerECD1"=w40:path, "DateinameECD1"=w39:string, "DateiordnerECD2"=w38:path, "DateinameECD2"=w37:string, "NamenLangsameHeizungen"=w35:string[], "ModuleLH"=w34:i32[])
      n7 = property on="AIsLH" class="Arr (strikt)"("Value"=w77) -> ()  [unwired: 2 in, 2 out]
      n8 = property on="ModuleLH" class="Arr (strikt)"("Value"=w34) -> ()  [unwired: 2 in, 2 out]
      n9 = property on="DIOsMod2BNr" class="Arr (strikt)"("Value"=w78) -> ()  [unwired: 2 in, 2 out]
      n10 = property on="AnzahlRegler/Modul" class="Arr (strikt)"("Value"=w76) -> ()  [unwired: 2 in, 2 out]
      n11 = property on="Regler für den Probenfluß" class="DigWert (strikt)"("Value"=w75) -> ()  [unwired: 2 in, 2 out]
      n12 = property on="DIOsMod0Nr" class="Arr (strikt)"("Value"=w81) -> ()  [unwired: 2 in, 2 out]
      n13 = property on="SPvorgebenMod0" class="Arr (strikt)"("Value"=w74) -> ()  [unwired: 2 in, 2 out]
      n14 = property on="DIOsMod1Nr" class="Arr (strikt)"("Value"=w80) -> ()  [unwired: 2 in, 2 out]
      n15 = property on="DIOsMod2ANr" class="Arr (strikt)"("Value"=w79) -> ()  [unwired: 2 in, 2 out]
      n16 = property on="ReglerNameMod2B" class="Arr (strikt)"("Value"=w44) -> ()  [unwired: 2 in, 2 out]
      n17 = property on="Startmethode" class="DigWert (strikt)"("Value"=w43) -> ()  [unwired: 2 in, 2 out]
      n18 = property on="Dateiordner Housekeeping" class="Pfad"("Value"=w42) -> ()  [unwired: 2 in, 2 out]
      n19 = property on="Dateiname Housekeeping" class="Str"("Value"=w41) -> ()  [unwired: 2 in, 2 out]
      n20 = property on="DateiordnerECD1" class="Pfad"("Value"=w40) -> ()  [unwired: 2 in, 2 out]
      n21 = property on="DateinameECD1" class="Str"("Value"=w39) -> ()  [unwired: 2 in, 2 out]
      n22 = property on="DateiordnerECD2" class="Pfad"("Value"=w38) -> ()  [unwired: 2 in, 2 out]
      n23 = property on="DateinameECD2" class="Str"("Value"=w37) -> ()  [unwired: 2 in, 2 out]
      n24 = property on="NamenLangsameHeizungen" class="Arr (strikt)"("Value"=w35) -> ()  [unwired: 2 in, 2 out]
      n25 = property on="SPvorgebenMod1" class="Arr (strikt)"("Value"=w73) -> ()  [unwired: 2 in, 2 out]
      n26 = property on="SPvorgebenMod2A" class="Arr (strikt)"("Value"=w72) -> ()  [unwired: 2 in, 2 out]
      n27 = property on="SPvorgebenMod2B" class="Arr (strikt)"("Value"=w71) -> ()  [unwired: 2 in, 2 out]
      n28 = property on="MWAntwortMod0" class="Arr (strikt)"("Value"=w70) -> ()  [unwired: 2 in, 2 out]
      n29 = property on="MWAntwortMod1" class="Arr (strikt)"("Value"=w69) -> ()  [unwired: 2 in, 2 out]
      n30 = property on="MWAntwortMod2A" class="Arr (strikt)"("Value"=w68) -> ()  [unwired: 2 in, 2 out]
      n31 = property on="MWAntwortMod2B" class="Arr (strikt)"("Value"=w67) -> ()  [unwired: 2 in, 2 out]
      n32 = property on="FaktorMod0" class="Arr (strikt)"("Value"=w66) -> ()  [unwired: 2 in, 2 out]
      n33 = property on="FaktorMod2B" class="Arr (strikt)"("Value"=w63) -> ()  [unwired: 2 in, 2 out]
      n34 = property on="MWabfragenMod0" class="Arr (strikt)"("Value"=w62) -> ()  [unwired: 2 in, 2 out]
      n35 = property on="FaktorMod1" class="Arr (strikt)"("Value"=w65) -> ()  [unwired: 2 in, 2 out]
      n36 = property on="MWabfragenMod1" class="Arr (strikt)"("Value"=w61) -> ()  [unwired: 2 in, 2 out]
      n37 = property on="FaktorMod2A" class="Arr (strikt)"("Value"=w64) -> ()  [unwired: 2 in, 2 out]
      n38 = property on="MWabfragenMod2A" class="Arr (strikt)"("Value"=w60) -> ()  [unwired: 2 in, 2 out]
      n39 = property on="MWabfragenMod2B" class="Arr (strikt)"("Value"=w59) -> ()  [unwired: 2 in, 2 out]
      n40 = property on="Modul1/AI koeff" class="Arr (strikt)"("Value"=w58) -> ()  [unwired: 2 in, 2 out]
      n41 = property on="Modul3/AI koeff" class="Arr (strikt)"("Value"=w56) -> ()  [unwired: 2 in, 2 out]
      n42 = property on="Traps/MachsKoeff" class="Arr (strikt)"("Value"=w55) -> ()  [unwired: 2 in, 2 out]
      n43 = property on="Modul1/AIsNamen" class="Arr (strikt)"("Value"=w54) -> ()  [unwired: 2 in, 2 out]
      n44 = property on="Modul2/AIsNamen" class="Arr (strikt)"("Value"=w53) -> ()  [unwired: 2 in, 2 out]
      n45 = property on="Modul3/AIsNamen" class="Arr (strikt)"("Value"=w52) -> ()  [unwired: 2 in, 2 out]
      n46 = property on="DIOsMod0Name" class="Arr (strikt)"("Value"=w51) -> ()  [unwired: 2 in, 2 out]
      n47 = property on="Modul2/AI koeff" class="Arr (strikt)"("Value"=w57) -> ()  [unwired: 2 in, 2 out]
      n48 = property on="DIOsMod1Name" class="Arr (strikt)"("Value"=w50) -> ()  [unwired: 2 in, 2 out]
      n49 = property on="DIOsMod2AName" class="Arr (strikt)"("Value"=w49) -> ()  [unwired: 2 in, 2 out]
      n50 = property on="DIOsMod2BName" class="Arr (strikt)"("Value"=w48) -> ()  [unwired: 2 in, 2 out]
      n51 = property on="ReglerNameMod0" class="Arr (strikt)"("Value"=w47) -> ()  [unwired: 2 in, 2 out]
      n52 = property on="ReglerNameMod1" class="Arr (strikt)"("Value"=w46) -> ()  [unwired: 2 in, 2 out]
      n53 = property on="ReglerNameMod2A" class="Arr (strikt)"("Value"=w45) -> ()  [unwired: 2 in, 2 out]
      "Schnelle Heizungen" <- string[] ["U_WiderstandTrap1", "U_TemperaturTrap1", "U_WiderstandTrap2", "U_TemperaturTrap2", "U_TemperaturMach1", "U_TemperaturMach2"]
    }
    frame #1 {
      n54 = while {
        tunnel: ["DIOsMod0Name"] -> w102
        tunnel: ["DIOsMod1Name"] -> w101
        tunnel: ["DIOsMod2AName"] -> w100
        tunnel: ["DIOsMod2BName"] -> w99
        tunnel: ["ReglerNameMod0"] -> w98
        tunnel: ["ReglerNameMod1"] -> w97
        tunnel: ["ReglerNameMod2A"] -> w96
        tunnel: ["ReglerNameMod2B"] -> w95
        tunnel: [w110] -> w94
        tunnel: ["ReglerNameMod2B"] -> w93
        tunnel: ["ReglerNameMod2A"] -> w92
        tunnel: ["ReglerNameMod1"] -> w91
        tunnel: ["ReglerNameMod0"] -> w90
        tunnel: ["DIOsMod0Name"] -> w88
        tunnel: ["DIOsMod1Name"] -> w87
        tunnel: ["DIOsMod2AName"] -> w86
        tunnel: ["DIOsMod2BName"] -> w85
        tunnel: ["NamenLangsameHeizungen"] -> w84
        tunnel: w83 -> [w105]
        stop <- "EinstellungenFertig" stop-if-true
        n55 = Wait (ms)(milliseconds to wait=u32 500 ("Zu wartende ms")) -> ()  [unwired: 1 out]
        n56 = case shown="True" "AIsNamenZurücksetzen" {
          frame False {
          }
          frame True {
            w176 = 32 ("Länge")
            w177 = string[] ["Mod1/AI0", "Mod1/AI1", "Mod1/AI2", "Mod1/AI3", "Mod1/AI4", "Mod1/AI5", "Mod1/AI6", "Mod1/AI7", "Mod1/AI8", "Mod1/AI9", "Mod1/AI10", "Mod1/AI11", "Mod1/AI12", "Mod1/AI13", "Mod1/AI14", "Mod1/AI15", "Mod1/AI16", "Mod1/AI17", "Mod1/AI18", "Mod1/AI19", "Mod1/AI20", "Mod1/AI21", "Mod1/AI22", "Mod1/AI23", "Mod1/AI24", "Mod1/AI25", "Mod1/AI26", "Mod1/AI27", "Mod1/AI28", "Mod1/AI29", "Mod1/AI30", "Mod1/AI31", "Mod2/AI0", "Mod2/AI1", "Mod2/AI2", "Mod2/AI3", "Mod2/AI4", "Mod2/AI5", "Mod2/AI6", "Mod2/AI7", "Mod2/AI8", "Mod2/AI9", "Mod2/AI10", "Mod2/AI11", "Mod2/AI12", "Mod2/AI13", "Mod2/AI14", "Mod2/AI15", "Mod2/AI16", "Mod2/AI17", "Mod2/AI18", "Mod2/AI19", "Mod2/AI20", "Mod2/AI21", "Mod2/AI22", "Mod2/AI23", "Mod2/AI24", "Mod2/AI25", "Mod2/AI26", "Mod2/AI27", "Mod2/AI28", "Mod2/AI29", "Mod2/AI30", "Mod2/AI31", "Mod3/AI0", "Mod3/AI1", "Mod3/AI2", "Mod3/AI3", "Mod3/AI4", "Mod3/AI5", "Mod3/AI6", "Mod3/AI7", "Mod3/AI8", "Mod3/AI9", "Mod3/AI10", "Mod3/AI11", "Mod3/AI12", "Mod3/AI13", "Mod3/AI14", "Mod3/AI15", "Mod3/AI16", "Mod3/AI17", "Mod3/AI18", "Mod3/AI19", "Mod3/AI20", "Mod3/AI21", "Mod3/AI22", "Mod3/AI23", "Mod3/AI24", "Mod3/AI25", "Mod3/AI26", "Mod3/AI27", "Mod3/AI28", "Mod3/AI29", "Mod3/AI30", "Mod3/AI31"] ("Array 2")
            n57 = Array Subset(array=w177, index=32 ("Index"), length=w176) -> (w173:string[])
            n58 = Array Subset(array=w177, index=0 ("Index"), length=w176) -> (w174:string[])
            n59 = Array Subset(array=w177, index=64 ("Index"), length=w176) -> (w172:string[])
            n60 = local write "Modul2/AIsNamen"(w173) -> ()
            n61 = local write "Modul1/AIsNamen"(w174) -> ()
            n62 = local write "Modul3/AIsNamen"(w172) -> ()
          }
        }
        n63 = Array Size(array="ReglerNameMod0") -> (size(s)=w160:i32)
        n64 = Array Size(array="ReglerNameMod1") -> (size(s)=w159:i32)
        n65 = Array Size(array="ReglerNameMod2A") -> (size(s)=w158:i32)
        n66 = Array Size(array="ReglerNameMod2B") -> (size(s)=w157:i32)
        n67 = Build Array "Anzahl Horst/Modul"(w160, w159, w158, w157) -> (w109:i32[])
        n68 = flat-sequence {
          tunnel: w109 -> [w170]
          tunnel: [w171] -> w108
          frame #0 {
            "AnzahlRegler/Modul" <- w170
          }
          frame #1 {
            n69 = local read "AnzahlRegler/Modul"() -> (w171:i32[])
          }
        }
        n70 = Build Array (concatenate)("Modul1/AIsNamen", "Modul2/AIsNamen", "Modul3/AIsNamen") -> (w110:string[])
        n71 = Bundle("DIOsMod0Nr"="DIOsMod0Nr", "DIOsMod1Nr"="DIOsMod1Nr", "DIOsMod2ANr"="DIOsMod2ANr", "DIOsMod2BNr"="DIOsMod2BNr", "AIsLH"="AIsLH", "AnzahlRegler/Modul"=w108, "Regler für den Probenfluß"="Regler für den Probenfluß", "SPvorgebenMod0"="SPvorgebenMod0", "SPvorgebenMod1"="SPvorgebenMod1", "SPvorgebenMod2A"="SPvorgebenMod2A", "SPvorgebenMod2B"="SPvorgebenMod2B", "MWAntwortMod0"="MWAntwortMod0", "MWAntwortMod1"="MWAntwortMod1", "MWAntwortMod2A"="MWAntwortMod2A", "MWAntwortMod2B"="MWAntwortMod2B", "FaktorMod0"="FaktorMod0", "FaktorMod1"="FaktorMod1", "FaktorMod2A"="FaktorMod2A", "FaktorMod2B"="FaktorMod2B", "MWabfragenMod0"="MWabfragenMod0", "MWabfragenMod1"="MWabfragenMod1", "MWabfragenMod2A"="MWabfragenMod2A", "MWabfragenMod2B"="MWabfragenMod2B", "Modul1/AI koeff"="Modul1/AI koeff", "Modul2/AI koeff"="Modul2/AI koeff", "Modul3/AI koeff"="Modul3/AI koeff", "Traps/MachsKoeff"="Traps/MachsKoeff", "Modul1/AIsNamen"="Modul1/AIsNamen", "Modul2/AIsNamen"="Modul2/AIsNamen", "Modul3/AIsNamen"="Modul3/AIsNamen", "DIOsMod0Name"="DIOsMod0Name", "DIOsMod1Name"="DIOsMod1Name", "DIOsMod2AName"="DIOsMod2AName", "DIOsMod2BName"="DIOsMod2BName", "ReglerNameMod0"="ReglerNameMod0", "ReglerNameMod1"="ReglerNameMod1", "ReglerNameMod2A"="ReglerNameMod2A", "ReglerNameMod2B"="ReglerNameMod2B", "Startmethode"="Startmethode", "Dateiordner Housekeeping"="Dateiordner Housekeeping", "Dateiname Housekeeping"="Dateiname Housekeeping", "DateiordnerECD1"="DateiordnerECD1", "DateinameECD1"="DateinameECD1", "DateiordnerECD2"="DateiordnerECD2", "DateinameECD2"="DateinameECD2", "NamenLangsameHeizungen"="NamenLangsameHeizungen", "ModuleLH"="ModuleLH") -> (w104:T8)  [unwired: 1 in]
        n72 = case shown="True" "EinstellungenSpeichern" {
          tunnel: w105 -> [_ w166]
          tunnel: w104 -> [_ w165]
          frame False {
          }
          frame True {
            n73 = Open/Create/Replace File(file path (use dialog)=w166, operation (0:open)=T7."replace" ("Operation (0:Öffnen)")) -> (refnum out=w168:refnum<file>, error out=w164:errorcluster)  [unwired: 4 in, 1 out]
            n74 = Write to Binary File(file (use dialog)=w168, data=w165, error in=w164) -> (refnum out=w167:refnum<file>, error out=w163:errorcluster)  [unwired: 3 in, 1 out]
            n75 = Close File(refnum=w167, error in=w163) -> (error out=w162:errorcluster)  [unwired: 1 out]
            n76 = call <vilib>:"Simple Error Handler.vi"("error in (no error)"=w162) -> ()  [unwired: 4 in, 5 out]
          }
        }
      }
      n77 = Build Array (concatenate)(w90, w91, w92, w93) -> (w89:string[])
    }
    frame #2 {
      w183 = string[] ["<", "<=", "=", ">=", ">", "=/="] ("Strings []")
      n78 = Build Array (concatenate)(w193, w192, w191, w190) -> (w188:string[])
      n79 = Build Array (concatenate)(w188, string[] ["ServoTrap1kalt", "ServoTrap2kalt", "Heizen?Trap1", "Heizen?Trap2", "Heizen?Mach1", "Heizen?Mach2", "Methodennummer", "STOPP!!!", "LHHorst1Heizen?", "LHMainCol1Heizen?", "LHMainCol2Heizen?", "LHHorst2Heizen?", "LHOvenHeizen?", "LHT-LineHeizen?"], w186) -> (w185:string[])
      n80 = Build Array (concatenate)(w195, string[] ["WiderstTrap1", "TempTrap1", "WiderstTrap2", "TempTrap2", "TempMach1", "TempMach2"], w186) -> (w184:string[])
      n81 = property on="AbfragbareVariablen2" class="Ring (strikt)"("Strings []"=w184) -> ()  [unwired: 2 in, 2 out]
      n82 = property on="BedienbareVariablen" class="Ring (strikt)"("Strings []"=w185) -> ()  [unwired: 2 in, 2 out]
      n83 = property on="AbfragbareVariablen1" class="Ring (strikt)"("Strings []"=w184) -> ()  [unwired: 2 in, 2 out]
      n84 = property on="Vergleichsoperator1" class="Ring (strikt)"("Strings []"=w183) -> ()  [unwired: 2 in, 2 out]
      n85 = property on="Vergleichsoperator2" class="Ring (strikt)"("Strings []"=w183) -> ()  [unwired: 2 in, 2 out]
      n86 = while {
        tunnel: w203 -> [w264]
        tunnel: w202 -> [w263]
        tunnel: w201 -> [w262]
        tunnel: w200 -> [w261]
        tunnel: w199 -> [w260]
        tunnel: w198 -> [w259]
        tunnel: w197 -> [w258]
        tunnel: w196 -> [w257]
        shift-right: [w214] -> w182
        shift-left: w189 -> [w253]
        tunnel: w184 -> [w221]
        tunnel: w183 -> [w220]
        tunnel: w185 -> [w219]
        tunnel: w180 -> [w213]
        stop <- w254 stop-if-true
        n87 = Index Array(array=w253, index="Methode Nummer") -> (element=w251:T9)
        n88 = Unbundle(w251) -> ("Zykluslängen [s]"=w250:dbl[], "ZeitpktDIOsMod0"=w249:dbl[], "ZeitpktDIOsMod1"=w248:dbl[], "ZeitpktDIOsMod2A"=w247:dbl[], "ZeitpktDIOsMod2B"=w246:dbl[], "DIOsSPMod0"=w245:bool[][], "DIOsSPMod1"=w244:bool[][], "DIOsSPMod2A"=w243:bool[][], "DIOsSPMod2B"=w242:bool[][], "Mod0HorstZeitpkt"=w241:dbl[], "Mod1HorstZeitpkt"=w240:dbl[], "Mod2AHorstZeitpkt"=w239:dbl[], "Mod2BHorstZeitpkt"=w238:dbl[], "HorstSPMod0"=w237:dbl[][], "HorstSPMod1"=w236:dbl[][], "HorstSPMod2A"=w235:dbl[][], "HorstSPMod2B"=w234:dbl[][], "LangsameHeizungenSP"=w233:dbl[], "LHHeizen?"=w232:bool[], "ZPktFPGABoolesch"=w231:dbl[], "FPGABoolesch"=w230:bool[][], "ZeitpktFPGAPID"=w229:dbl[], "FPGAPID"=w228:T3, "ZeitpktFPGAFixp"=w227:dbl[], "FPGAFixp"=w226:fxp<+/-,16,4>[][], "ZeitpktMach1"=w225:dbl[], "TempMach1"=w224:dbl[], "ZeitpktMach2"=w223:dbl[], "TempMach2"=w222:dbl[], "PIDs für \"träge\" Heizungen"=w218:T2, "Zwangsbedingungen"=w217:dbl[][], "Dateien fürs MS schicken?"=w216:bool, "ZeitpunkteMPV"=w209:dbl[], "SPMPV"=w208:i32[], "ZeitpktMSa"=w211:dbl, "ZeitpktMSb"=w210:dbl, "Int.Start1"=w207:dbl, "Int.Stop1"=w206:dbl, "Int.Start2"=w205:dbl, "Int.Stop2"=w204:dbl, "Methodenname"=w212:string)
        n89 = property on="ZeitpktMS-2" class="DigWert (strikt)"("Value"=w210) -> ()  [unwired: 2 in, 2 out]
        n90 = property on="ZeitpktMS-1" class="DigWert (strikt)"("Value"=w211) -> ()  [unwired: 2 in, 2 out]
        n91 = property on="Methodenname" class="Str"("Value"=w212) -> ()  [unwired: 2 in, 2 out]
        n92 = property on="Int.Stop2" class="DigWert (strikt)"("Value"=w204) -> ()  [unwired: 2 in, 2 out]
        n93 = property on="Int.Stop1" class="DigWert (strikt)"("Value"=w206) -> ()  [unwired: 2 in, 2 out]
        n94 = property on="Int.Start2" class="DigWert (strikt)"("Value"=w205) -> ()  [unwired: 2 in, 2 out]
        n95 = property on="ZeitpunkteMPV" class="Arr (strikt)"("Value"=w209) -> ()  [unwired: 2 in, 2 out]
        n96 = property on="SPMPV" class="Arr (strikt)"("Value"=w208) -> ()  [unwired: 2 in, 2 out]
        n97 = property on="Int.Start1" class="DigWert (strikt)"("Value"=w207) -> ()  [unwired: 2 in, 2 out]
        n98 = property on="LHHeizen?" class="Arr (strikt)"("Value"=w232) -> ()  [unwired: 2 in, 2 out]
        n99 = property on="FPGAPID" class="Arr (strikt)"("Value"=w228) -> ()  [unwired: 2 in, 2 out]
        n100 = property on="FPGAFixp" class="Arr (strikt)"("Value"=w226) -> ()  [unwired: 2 in, 2 out]
        n101 = property on="Zykluslängen [s]" class="Arr (strikt)"("Value"=w250) -> ()  [unwired: 2 in, 2 out]
        n102 = property on="ZeitpktDIOsMod0" class="Arr (strikt)"("Value"=w249) -> ()  [unwired: 2 in, 2 out]
        n103 = property on="Mod2BHorstZeitpkt" class="Arr (strikt)"("Value"=w238) -> ()  [unwired: 2 in, 2 out]
        n104 = property on="HorstSPMod0" class="Arr (strikt)"("Value"=w237) -> ()  [unwired: 2 in, 2 out]
        n105 = property on="LHSetpoints" class="Arr (strikt)"("Value"=w233) -> ()  [unwired: 2 in, 2 out]
        n106 = property on="ZPktFPGABoolesch" class="Arr (strikt)"("Value"=w231) -> ()  [unwired: 2 in, 2 out]
        n107 = property on="FPGABoolesch" class="Arr (strikt)"("Value"=w230) -> ()  [unwired: 2 in, 2 out]
        n108 = property on="TempMach2" class="Arr (strikt)"("Value"=w222) -> ()  [unwired: 2 in, 2 out]
        n109 = property on="PIDs für \"träge\" Heizungen" class="Arr (strikt)"("Value"=w218) -> ()  [unwired: 2 in, 2 out]
        n110 = property on="DIOsSPMod1" class="Arr (strikt)"("Value"=w244) -> ()  [unwired: 2 in, 2 out]
        n111 = property on="DIOsSPMod2A" class="Arr (strikt)"("Value"=w243) -> ()  [unwired: 2 in, 2 out]
        n112 = property on="HorstSPMod1" class="Arr (strikt)"("Value"=w236) -> ()  [unwired: 2 in, 2 out]
        n113 = property on="HorstSPMod2A" class="Arr (strikt)"("Value"=w235) -> ()  [unwired: 2 in, 2 out]
        n114 = property on="HorstSPMod2B" class="Arr (strikt)"("Value"=w234) -> ()  [unwired: 2 in, 2 out]
        n115 = property on="ZeitpktFPGAPID" class="Arr (strikt)"("Value"=w229) -> ()  [unwired: 2 in, 2 out]
        n116 = property on="ZeitpktFPGAFixp" class="Arr (strikt)"("Value"=w227) -> ()  [unwired: 2 in, 2 out]
        n117 = property on="ZeitpktMach1" class="Arr (strikt)"("Value"=w225) -> ()  [unwired: 2 in, 2 out]
        n118 = property on="TempMach1" class="Arr (strikt)"("Value"=w224) -> ()  [unwired: 2 in, 2 out]
        n119 = property on="ZeitpktMach2" class="Arr (strikt)"("Value"=w223) -> ()  [unwired: 2 in, 2 out]
        n120 = property on="ZeitpktDIOsMod1" class="Arr (strikt)"("Value"=w248) -> ()  [unwired: 2 in, 2 out]
        n121 = property on="ZeitpktDIOsMod2A" class="Arr (strikt)"("Value"=w247) -> ()  [unwired: 2 in, 2 out]
        n122 = property on="ZeitpktDIOsMod2B" class="Arr (strikt)"("Value"=w246) -> ()  [unwired: 2 in, 2 out]
        n123 = property on="DIOsSPMod0" class="Arr (strikt)"("Value"=w245) -> ()  [unwired: 2 in, 2 out]
        n124 = property on="DIOsSPMod2B" class="Arr (strikt)"("Value"=w242) -> ()  [unwired: 2 in, 2 out]
        n125 = property on="Mod0HorstZeitpkt" class="Arr (strikt)"("Value"=w241) -> ()  [unwired: 2 in, 2 out]
        n126 = property on="Mod1HorstZeitpkt" class="Arr (strikt)"("Value"=w240) -> ()  [unwired: 2 in, 2 out]
        n127 = property on="Mod2AHorstZeitpkt" class="Arr (strikt)"("Value"=w239) -> ()  [unwired: 2 in, 2 out]
        n128 = property on="Dateien fürs MS schicken?" class="Bool. (strikt)"("Value"=w216) -> ()  [unwired: 2 in, 2 out]
        n129 = while {
          tunnel: w263 -> [w360]
          tunnel: w262 -> [w359]
          tunnel: w261 -> [w358]
          tunnel: w260 -> [w357]
          tunnel: w259 -> [w356]
          tunnel: w257 -> [w355]
          tunnel: w258 -> [w354]
          tunnel: w264 -> [w324]
          tunnel: [w323] -> w255
          tunnel: [w281] -> w256
          tunnel: ["EditorBeenden"] -> w254
          tunnel: w221 -> [w309]
          shift-right: [w304] -> _
          shift-left: w217 -> [w308]
          tunnel: w220 -> [w307]
          tunnel: w219 -> [w306]
          tunnel: ["AllesSpeichern"] -> w215
          stop <- w283 stop-if-true
          n130 = for {
            tunnel: w308 -> [w369] mode=indexing
            tunnel: w309 -> [w365]
            tunnel: w307 -> [w364]
            tunnel: w306 -> [w383]
            tunnel: [w377] -> w317 mode=indexing
            n131 = Index Array(array=w369, index=0 ("Index")) -> (element=w389:dbl)
            n132 = Index Array(array=w369, index=1 ("Index")) -> (element=w387:dbl)
            n133 = Index Array(array=w369, index=3 ("Index")) -> (element=w371:dbl)
            n134 = Index Array(array=w369, index=4 ("Index")) -> (element=w370:dbl)
            n135 = Index Array(array=w369, index=6 ("Index")) -> (element=w385:dbl)
            n136 = To Long Integer(number=w389) -> (32bit integer=w388:i32)
            n137 = To Long Integer(number=w387) -> (32bit integer=w386:i32)
            n138 = To Long Integer(number=w371) -> (32bit integer=w368:i32)
            n139 = To Long Integer(number=w370) -> (32bit integer=w367:i32)
            n140 = To Long Integer(number=w385) -> (32bit integer=w384:i32)
            n141 = Index Array(array=w369, index=2 ("Index")) -> (element=w382:dbl)
            n142 = Index Array(array=w369, index=5 ("Index")) -> (element=w366:dbl)
            n143 = Index Array(array=w369, index=7 ("Index")) -> (element=w381:dbl)
            n144 = Index Array(array=w365, index=w388) -> (element=w380:string)
            n145 = Index Array(array=w364, index=w386) -> (element=w379:string)
            n146 = Index Array(array=w365, index=w368) -> (element=w363:string)
            n147 = Index Array(array=w364, index=w367) -> (element=w362:string)
            n148 = Index Array(array=w383, index=w384) -> (element=w375:string)
            n149 = Number To Exponential String(number=w382) -> (E-format string=w378:string)  [unwired: 3 in]
            n150 = Number To Exponential String(number=w366) -> (E-format string=w361:string)  [unwired: 3 in]
            n151 = Number To Exponential String(number=w381) -> (E-format string=w376:string)  [unwired: 3 in]
            n152 = Build Array(w380, w379, w378, w363, w362, w361, w375, w376) -> (w377:string[])
          }
          "ZwangsBedingungen" <- w317
          n153 = Wait (ms)(milliseconds to wait=u32 500 ("Zu wartende ms")) -> ()  [unwired: 1 out]
          n154 = call "Machmodul Spannung zu Temp (SubVI).vi"("Temp PT 100 soll"="Temperatur Mach") -> ("U soll"=→"Spannung Mach":fxp<+/-,16,4>)  [unwired: 1 in, 1 out]
          n155 = call "PT 100 Spannung zu Temp (SubVI).vi"("Temp PT 100 soll"="Temperatur Trap") -> ("U soll"=→"Spannung Trap":fxp<+/-,16,4>)  [unwired: 1 in, 1 out]
          n156 = Build Array("AbfragbareVariablen1", "Vergleichsoperator1", "Wert1", "AbfragbareVariablen2", "Vergleichsoperator2", "Wert2", "BedienbareVariablen", "Ausgangswert") -> (w314:dbl[])
          n157 = case shown="False" "Bedingung übernehmen" {
            tunnel: w308 -> [w399 w402]
            tunnel: w314 -> [_ w401]
            tunnel: [w399 w400] -> w315
            frame False {
            }
            frame True {
              n158 = Build Array (concatenate)(w402, w401) -> (w400:dbl[][])
            }
          }
          n159 = case shown="True" "löschen" {
            tunnel: w315 -> [w395 w398]
            tunnel: [w395 w396] -> w304
            frame False {
            }
            frame True {
              n160 = Delete From Array(array=w398, index (row)="Bedingung Nr. X") -> (array with subset deleted=w396:dbl[][])  [unwired: 2 in, 1 out]
            }
          }
          n161 = local write "Zwangsbedingungen"(w304) -> ()
          n162 = Or(x="MethodeSpeichern", y="EditorBeenden") -> (x .or. y?=w321:bool)
          n163 = Or(x=w321, y="MethodeLaden") -> (x .or. y?=w284:bool)
          n164 = Or(x=w284, y="AllesSpeichern") -> (x .or. y?=w283:bool)
          n165 = Or(x="AllesSpeichern", y="MethodeSpeichern") -> (x .or. y?=w281:bool)
          n166 = Bundle("Zykluslängen [s]"="Zykluslängen [s]", "ZeitpktDIOsMod0"="ZeitpktDIOsMod0", "ZeitpktDIOsMod1"="ZeitpktDIOsMod1", "ZeitpktDIOsMod2A"="ZeitpktDIOsMod2A", "ZeitpktDIOsMod2B"="ZeitpktDIOsMod2B", "DIOsSPMod0"="DIOsSPMod0", "DIOsSPMod1"="DIOsSPMod1", "DIOsSPMod2A"="DIOsSPMod2A", "DIOsSPMod2B"="DIOsSPMod2B", "Mod0HorstZeitpkt"="Mod0HorstZeitpkt", "Mod1HorstZeitpkt"="Mod1HorstZeitpkt", "Mod2AHorstZeitpkt"="Mod2AHorstZeitpkt", "Mod2BHorstZeitpkt"="Mod2BHorstZeitpkt", "HorstSPMod0"="HorstSPMod0", "HorstSPMod1"="HorstSPMod1", "HorstSPMod2A"="HorstSPMod2A", "HorstSPMod2B"="HorstSPMod2B", "LHSetpoints"="LHSetpoints", "LHHeizen?"="LHHeizen?", "ZPktFPGABoolesch"="ZPktFPGABoolesch", "FPGABoolesch"="FPGABoolesch", "ZeitpktFPGAPID"="ZeitpktFPGAPID", "FPGAPID"="FPGAPID", "ZeitpktFPGAFixp"="ZeitpktFPGAFixp", "FPGAFixp"="FPGAFixp", "ZeitpktMach1"="ZeitpktMach1", "TempMach1"="TempMach1", "ZeitpktMach2"="ZeitpktMach2", "TempMach2"="TempMach2", "PIDs für \"träge\" Heizungen"="PIDs für \"träge\" Heizungen", "Zwangsbedingungen"="Zwangsbedingungen", "Dateien fürs MS schicken?"="Dateien fürs MS schicken?", "ZeitpunkteMPV"="ZeitpunkteMPV", "SPMPV"="SPMPV", "ZeitpktMS-1"="ZeitpktMS-1", "ZeitpktMS-2"="ZeitpktMS-2", "Int.Start1"="Int.Start1", "Int.Stop1"="Int.Stop1", "Int.Start2"="Int.Start2", "Int.Stop2"="Int.Stop2", "Methodenname"="Methodenname") -> (w323:T10)  [unwired: 1 in]
          "DIOsMod0Name" <- w324
          "DIOsMod1Name" <- w360
          "DIOsMod2AName" <- w359
          "DIOsMod2BName" <- w358
          "HorstMod0Name" <- w357
          "HorstMod2BName" <- w354
          "HorstMod2AName" <- w355
          "HorstMod1Name" <- w356
        }
        n167 = case shown="True" w256 {
          tunnel: w253 -> [w273 w279]
          tunnel: w255 -> [_ w274]
          tunnel: [w273 w275] -> w214
          tunnel: "Methode Nummer" -> [_ w276]
          frame False {
          }
          frame True {
            n168 = Delete From Array(array=w279, length=1 ("Länge"), index=w276) -> (array with subset deleted=w277:T1)  [unwired: 1 out]
            n169 = Insert Into Array(array=w277, index=w276, new element=w274) -> (w275:T1)
          }
        }
        n170 = case shown="True" w215 {
          tunnel: w214 -> [_ w270]
          tunnel: w213 -> [_ w265]
          frame False {
          }
          frame True {
            n171 = Open/Create/Replace File(file path (use dialog)=w265, operation (0:open)=T7."replace" ("Operation (0:Öffnen)")) -> (refnum out=w269:refnum<file>, error out=w271:errorcluster)  [unwired: 4 in, 1 out]
            n172 = Write to Binary File(file (use dialog)=w269, data=w270, error in=w271) -> (refnum out=w267:refnum<file>, error out=w268:errorcluster)  [unwired: 3 in, 1 out]
            n173 = Close File(refnum=w267, error in=w268) -> (error out=w266:errorcluster)  [unwired: 1 out]
            n174 = call <vilib>:"Simple Error Handler.vi"("error in (no error)"=w266) -> ()  [unwired: 4 in, 5 out]
          }
        }
      }
      "Methoden" <- w182
      "LangsameHeizungen" <- w181
    }
  }
  n175 = Open/Create/Replace File(file path (use dialog)=path "C:/methoden.per" ("Dateipfad Methoden")) -> (refnum out=w8:refnum<file>, error out=w7:errorcluster)  [unwired: 5 in, 1 out]
  n176 = Read from Binary File(5:T1 [], 8:w7, 11:w8) -> (0:w3:errorcluster, 2:w6:T1, 3:w4:refnum<file>)  [unwired: 3 in, 1 out]
  n177 = Close File(refnum=w4, error in=w3) -> (path=w1:path, error out=w2:errorcluster)
  n178 = call <vilib>:"Simple Error Handler.vi"("error in (no error)"=w2) -> ()  [unwired: 4 in, 5 out]
